vi "SP_Auto_Read_Write.vi"() -> ()   [LabVIEW 2013]
uses:
  <vilib>/event_ctls.llb/eventvkey.ctl
  Global_Not-Aus.vi
  Global_Start_Stop_Einzelschritt.vi
  <vilib>/Utility/file.llb/Write To Spreadsheet File (DBL).vi
  <vilib>/Utility/file.llb/Read From Spreadsheet File (string).vi
panel:
  in  "Multiple Control":T1(tab)
  out "P6":dbl[](array[numeric])
  out "P5":dbl[](array[numeric])
  out "P4":dbl[](array[numeric])
  out "P3":dbl[](array[numeric])
  out "P7":dbl[](array[numeric])
  out "P2":dbl[](array[numeric])
  out "P1":dbl[](array[numeric])
  out "P8":dbl[](array[numeric])
  out "P9":dbl[](array[numeric])
  out "P10":dbl[](array[numeric])
  in  "Z axis":enum16{"Up", "Down"}(ring)
  in  "Y axis":enum16{"Forward", "Backward"}(ring)
  in  "X axis":enum16{"Left", "Right"}(ring)
  in  "Move Steps":bool
  in  "Steps(mm)":dbl[](array[numeric]) min=0.0
  in  "Go To":bool
  in  "Position":T2(ring)
  in  "Save":bool
  in  "Reset All":bool
  in  "Reset":bool
  in  "Import":bool
  in  "Export":bool
  in  "File Path":path=path "Y:/01_Projekte/EPN93031_Schreibplatz/8_Konstruktionsunterlagen/8.5_Software/COPY_KOSY Steuerung LabVIEW/1.New_Code_2014_2015/2Pole_strip_Position.txt"
  out "Speed":dbl(knob) scale=0.0..10.0
  in  "Port for KOSY3":refnum<visa-resource-name>="COM2"
  in  "Port for Powersupply":refnum<visa-resource-name>="COM3"
  in  "Port for Write Head":refnum<visa-resource-name>="COM4"
  in  "Port for ED33":refnum<visa-resource-name>="COM7"
  in  "Port for ED32i":refnum<visa-resource-name>="COM8"
  in  "X,Y,Z Value Limits":T3={"mm Xmin "=0.0, "mm Xmax "=100.0, " mm Ymin "=0.0, "mm Ymax "=267.9, " mm Zmin"=0.0, "mm Zmax "=108.0, "Schritte oder mm Umin (0)"=0.0, "Schritte oder mm Umax (0)"=0.0, "Schritte oder mm Cmin (0)"=0.0, "Schritte oder mm Cmax (0)"=0.0, "Schritte oder mm Amin (0)"=0.0, "Schritte oder mm Amax (0)"=0.0, "Schritte oder mm Bmin (0)"=0.0, "Schritte oder mm Bmax (0)"=0.0}
  out "Error Out":errorcluster caption="error out"
  in  "Error In":errorcluster caption="error in"
  out "Movement":T4={"Axis"=36, "Direction(To/From)"=0, "Speed in mm/s\n (5)[0,025-20]"=5.0, "IV6"=FALSE} {"Direction(To/From)" items=["vom Endschalter weg", "zum Endschalter hin"]; "Speed in mm/s\n (5)[0,025-20]" min=0.025 max=20; "Axis" items=["X-Achse"=36, "Y-Achse"=37, "Z-Achse"=38, "U-Achse"=63]}
  out "Keyboard Press Display":cluster{"Speed(+/-)":i16, "Movement":T5}
  in  "Count":dbl
  in  "Move & Measure":bool
  in  "Clear Sensor Readings":bool
  in  "ED32i Active?":bool
  in  "ED33 Active?":bool
  in  "Stop Program":bool
  in  "Instructions":enum32{"Page 2"}(tab)
  in  "Main Tab":enum32{"Page 1", "Page 2"}(tab)
  in  "File Select":enum32{"Page 1"}(tab)
  out "Steps":dbl
  out "Current Sequence":string[](array[string])
  in  "Clear Sequence":bool
  in  "Load Sequence":bool
  out "Sequence":string[][](array[string])
  in  "File  Select":path
  in  "Activate Sequence?":bool
  in  "Results":enum32{"Page 1"}(tab)
  out "ED32i":cluster{"Array 4[0]":i32, "Array 4[1]":i32}(graph)
  out "ED33":i32[](graph)
  out "ED32i_output":string[][](array[string])
  out "ED33_output":string[][](array[string])
  in  "Home Position":bool
  out "Operation Done":string="Initialise"
  out "Current Status":string="Initialise"
  out "Moving":bool
  out "Stopped":bool
  out "Current Cordinates":T6 {"Schritte B" format="%#.4g"; "Schritte A" format="%#.4g"; "Schritte C" format="%#.4g"; "Schritte U" format="%#.4g"; "Z axis" format="%#.4g"; "Y axis" format="%#.4g"; "X axis" format="%#.4g"}
  # "Polestrip Positions"
  # "Com port info"
  # "Waveform Dispaly"
  # "Instructions\n                                              Manual Control\n1. Run the program.\n2. Select 'Initialise' to start the program from first \n     or 'Continue' to continue the ongoing process.\n3. Select 'Normal Operation'.\n\nPolestrip Positions\n1. If already positions are already saved, select the corresponding \n    file in 'File Path' and then click 'Import' to get the corresponding\n    positions displayed on the front panel. \n2. Set the 'Speed' using (+/-) for the movement.\n3. Select a position from the dropdown 'Position'and click 'Go To'.\n    Else, \n1. Set the 'Speed' using (+/-) for the movement.\n2. Set the length for movement in 'Steps(mm)'  in corresponding \n    axis and also the direction of travel in the selected axis. \n    Then press 'Move'.\n3. Once desired position is reached, select a position from the \n    dropdown 'Position' and click 'Save'.\n4. Once all positions are saved in front panel, select the file  to be \n     saved in 'File Path' and click 'Export' to save positions to a text file.\n5. Select a position from the dropdown 'Position' and \n    Click 'Reset' to clear individual position.\n6. Click 'Reset All' to clear all positions.\n \nSensor Readings\nContinuous measurement\n1.Activate the sensor to be read from 'Read Sensors' tab.\n2.Set the length for movement in 'Steps(mm)' in corresponding \n    axis and also the direction of travel in the selected axis. \n    Then press 'Move'.\nMove and Measure\n1. Activate the sensor to be read from 'Read Sensors' tab.\n2.Set 'Count' to the number of times to measure.\n2.Set the length for movement in 'Steps(mm)' in corresponding \n    axis and also the direction of travel in the selected axis. \n    Then press 'Move Measure'.\n\n1. Click 'Clear' in 'Read Sensors' tab to clear the sensor readings.\n\n                                          Automatic Execution\n1. Run the program.\n2. Select 'Initialise' to start the program from first \n     or 'Continue' to continue the ongoing process.\n3. Select 'Normal Operation'.\n4. Select the corresponding file in 'File Select' and then click 'Load' \n    to get the corresponding codes in 'Sequence' .\n5. Click 'Clear' to clear sequence.\n6. Click 'Activate Sequence?' to run the automatic execution. \n\n                                                       General\n1. Click 'Stop Program' to stop the running program.\n2. Click 'Home Position' to take the write head to (0,0,0)."
  # "Instructions\n\n\n1. Select the corresponding file in 'File Select' \n    and click 'Load' to get the codes in\n    'Sequence'.\n2. Click 'Clear' to clear sequence.\n3. Click 'Activate Sequence?' to run\n     the automatic execution."
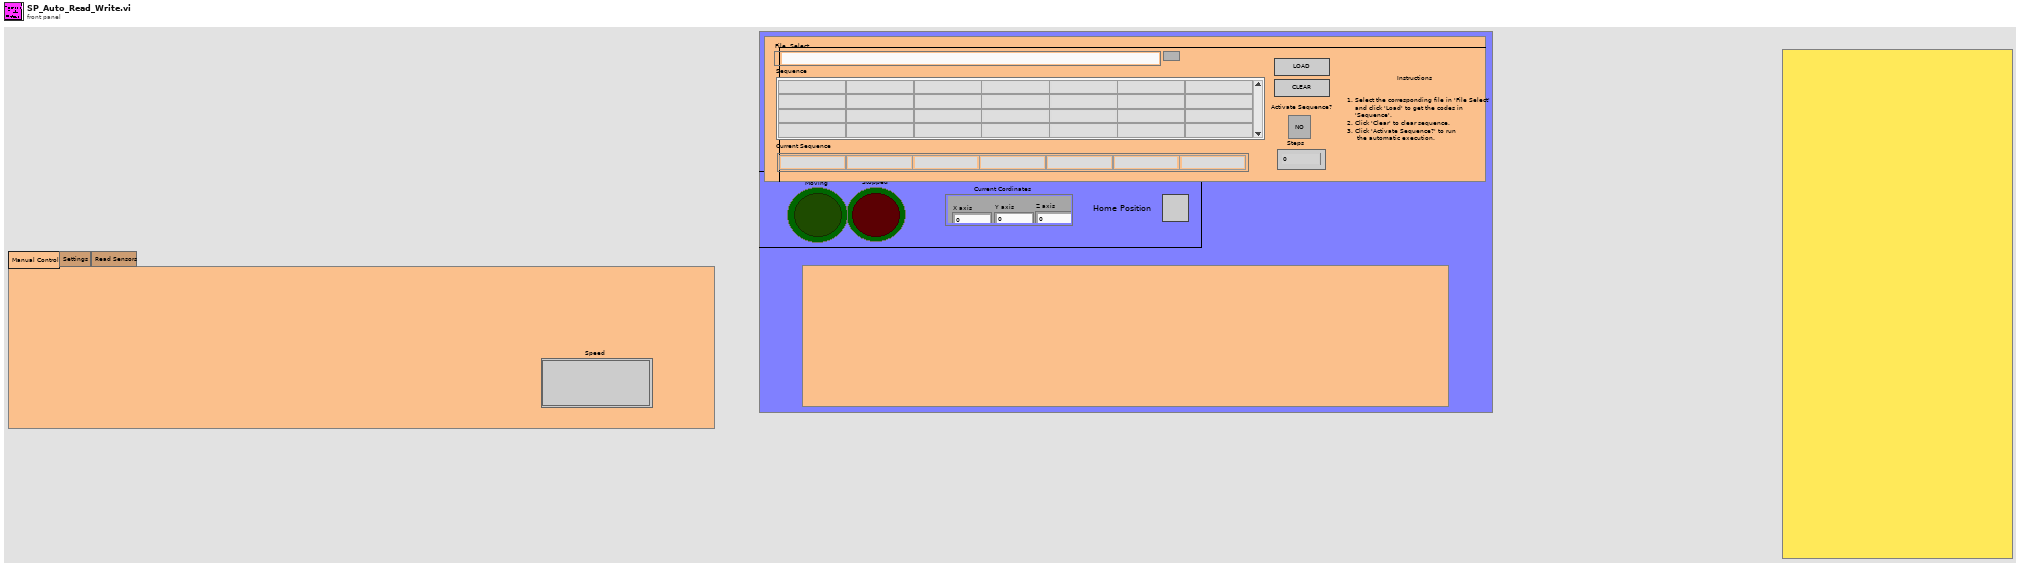
[diagram p1: front panel]
types:
  T1 = enum32{"Manual Control", "Settings", "Read Sensors"}
  T2 = enum16{"Position 1", "Position 2", "Position 3", "Position 4", "Position 5", "Position 6", "Position 7", "Position 8", "Position 9", "Position 10"}
  T3 = cluster{"mm Xmin ":sgl, "mm Xmax ":sgl, " mm Ymin ":sgl, "mm Ymax ":sgl, " mm Zmin":sgl, "mm Zmax ":sgl, "Schritte oder mm Umin (0)":sgl, "Schritte oder mm Umax (0)":sgl, "Schritte oder mm Cmin (0)":sgl, "Schritte oder mm Cmax (0)":sgl, "Schritte oder mm Amin (0)":sgl, "Schritte oder mm Amax (0)":sgl, "Schritte oder mm Bmin (0)":sgl, "Schritte oder mm Bmax (0)":sgl}
  T4 = cluster{"Axis":u8, "Direction(To/From)":u8, "Speed in mm/s\n (5)[0,025-20]":sgl, "IV6":bool}
  T5 = typedef "eventvkey.ctl" = enum16{"ASCII", "Enter", "Return", "Shift", "Ctrl", "Alt", "Cmd", "Opt", "Caps", "NumLock", "Clear", "Break", "Up", "Down", "Left", "Right", "Insert", "Delete", "Home", "End", "PageUp", "PageDown", "Escape", "Help", "Pause", "ScrollLock", "F1", "F2", "F3", "F4", "F5", "F6", "F7", "F8", "F9", "F10", "F11", "F12", "F13", "F14", "F15", "F16", "F17", "F18", "F19", "F20", "F21", "F22", "F23", "F24", "Play", "VolumeUp", "VolumeDown", "Mute", "Two Byte Char"}
  T6 = cluster{"X axis":sgl, "Y axis":sgl, "Z axis":sgl, "Schritte U":sgl, "Schritte C":sgl, "Schritte A":sgl, "Schritte B":sgl}
  T7 = enum32{"Page Enabled", "Page Disabled", "Page Disabled & Grayed"}
  T8 = cluster{"Geschwindigkeit X in mm/s\n(5) [0,025-15]":sgl, "Geschwindigkeit Y in mm/s\n(5) [0,025-15]":sgl, "Geschwindigkeit Z in mm/s\n(5) [0,025-15]":sgl, "GeschwindigkeitU in mm/s\n(5) [0,025-15]":sgl}
  T9 = cluster{"Schritte X":sgl, "Schritte Y":sgl, "Schritte Z":sgl, "Schritte U":sgl, "Schritte C":sgl, "Schritte A":sgl, "Schritte B":sgl}
  T10 = cluster{"[0]":dbl, "[1]":dbl, "[2]":dbl, "[3]":dbl, "[4]":dbl, "[5]":dbl, "[6]":dbl, "[7]":dbl, "[8]":dbl}
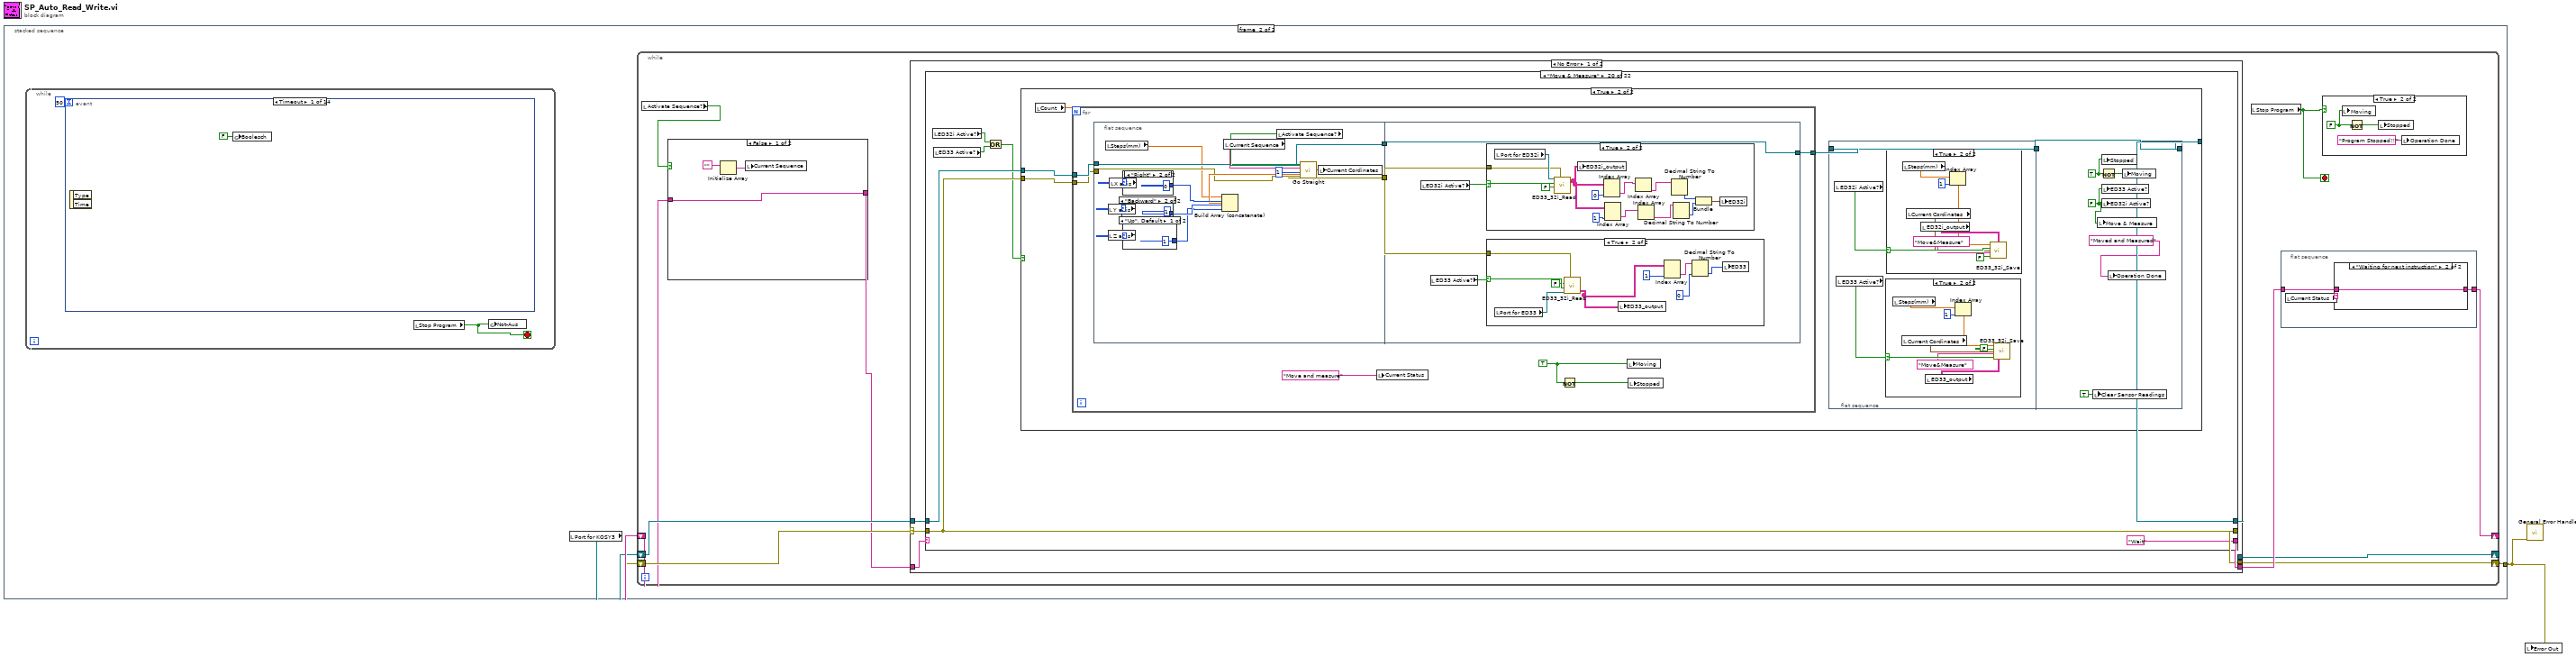
[diagram p0: block diagram]
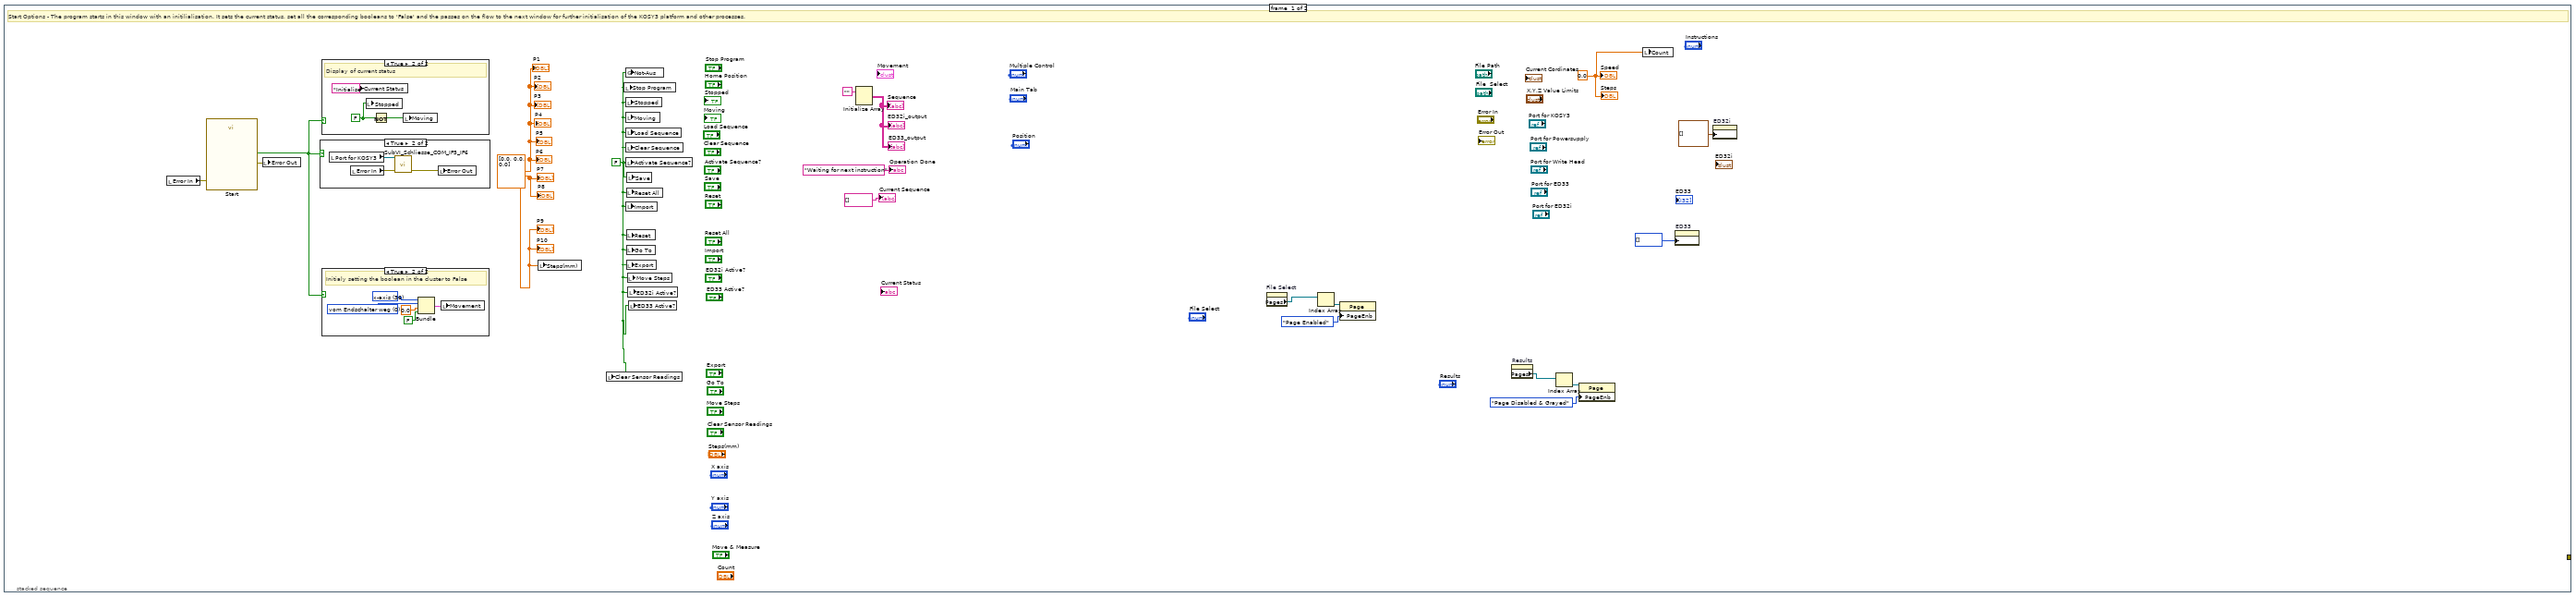
[diagram p2: hidden frame]
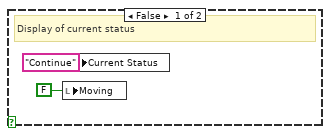
[diagram p5: hidden frame]
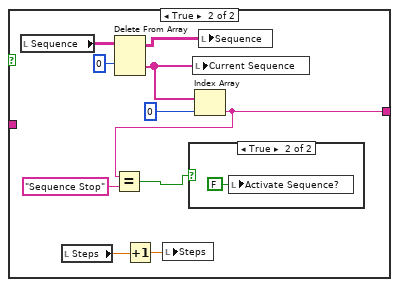
[diagram p6: hidden frame]
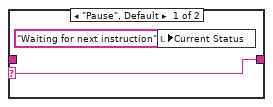
[diagram p9: hidden frame]
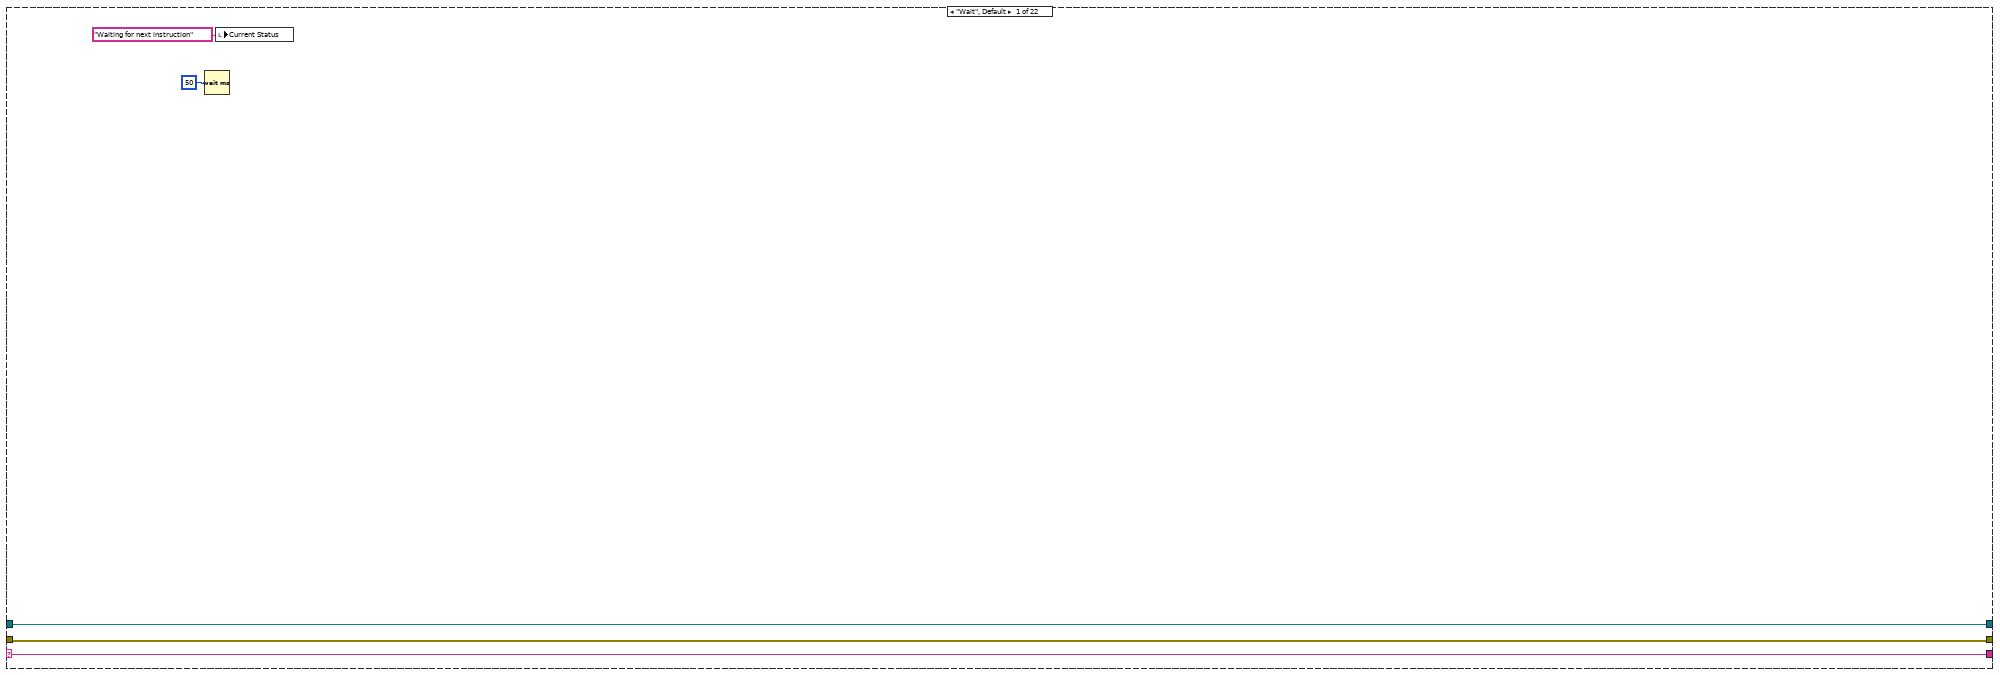
[diagram p10: hidden frame]
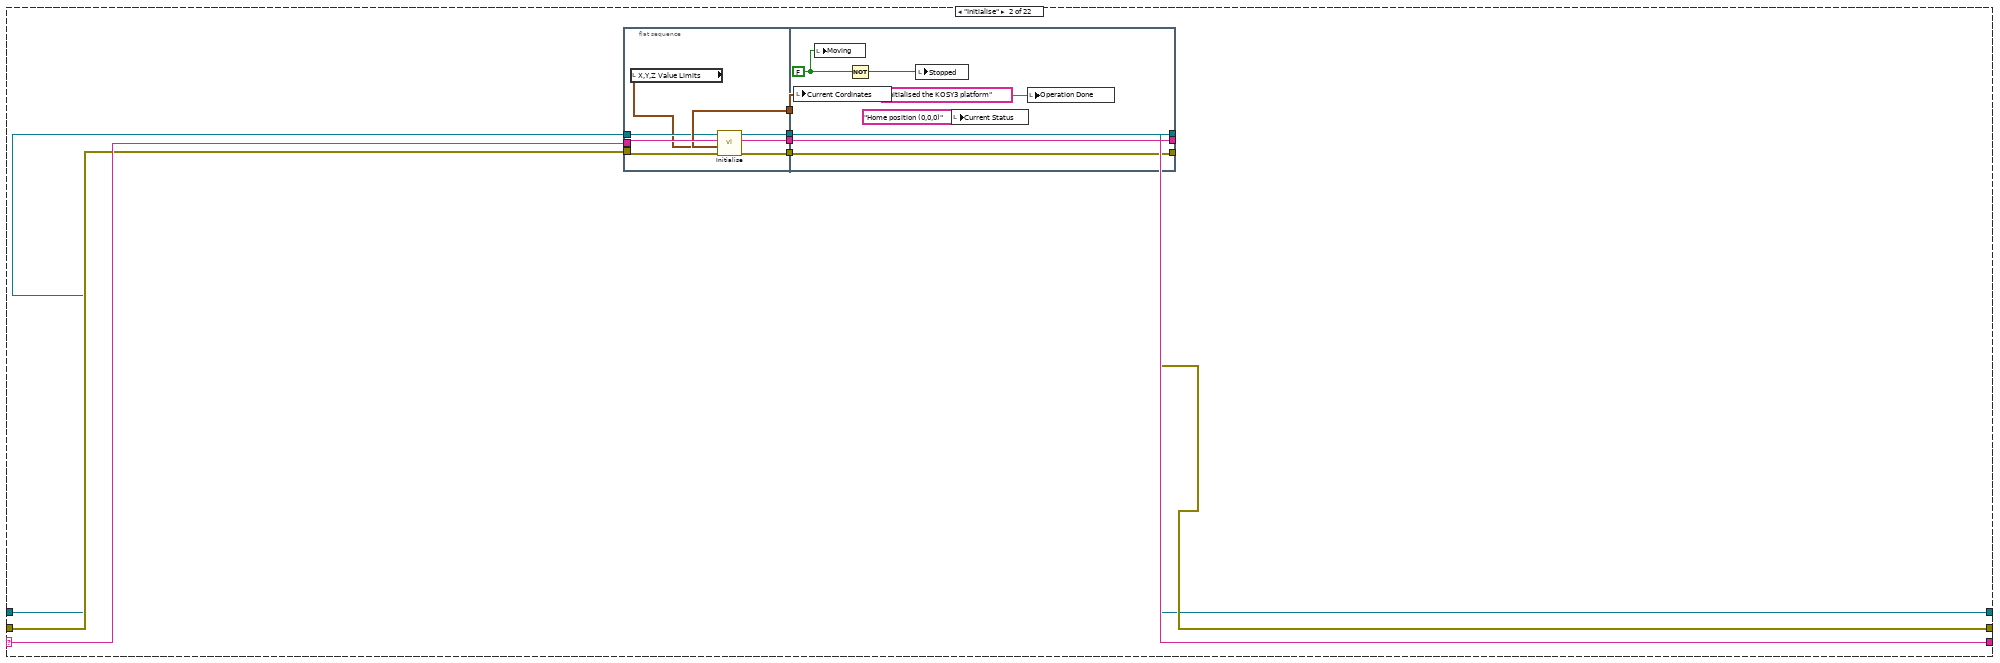
[diagram p11: hidden frame]
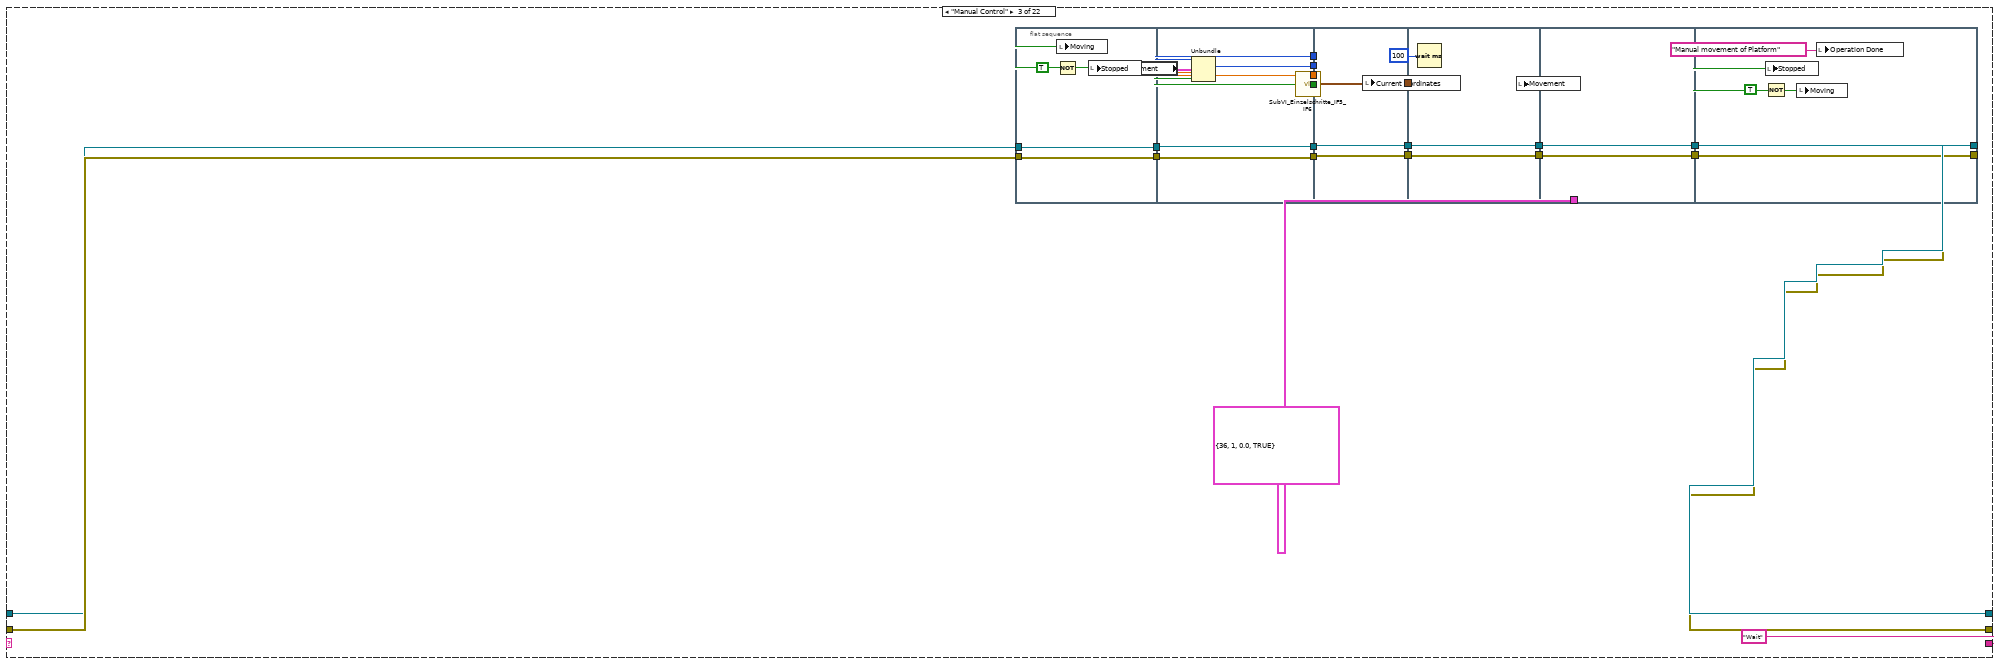
[diagram p12: hidden frame]
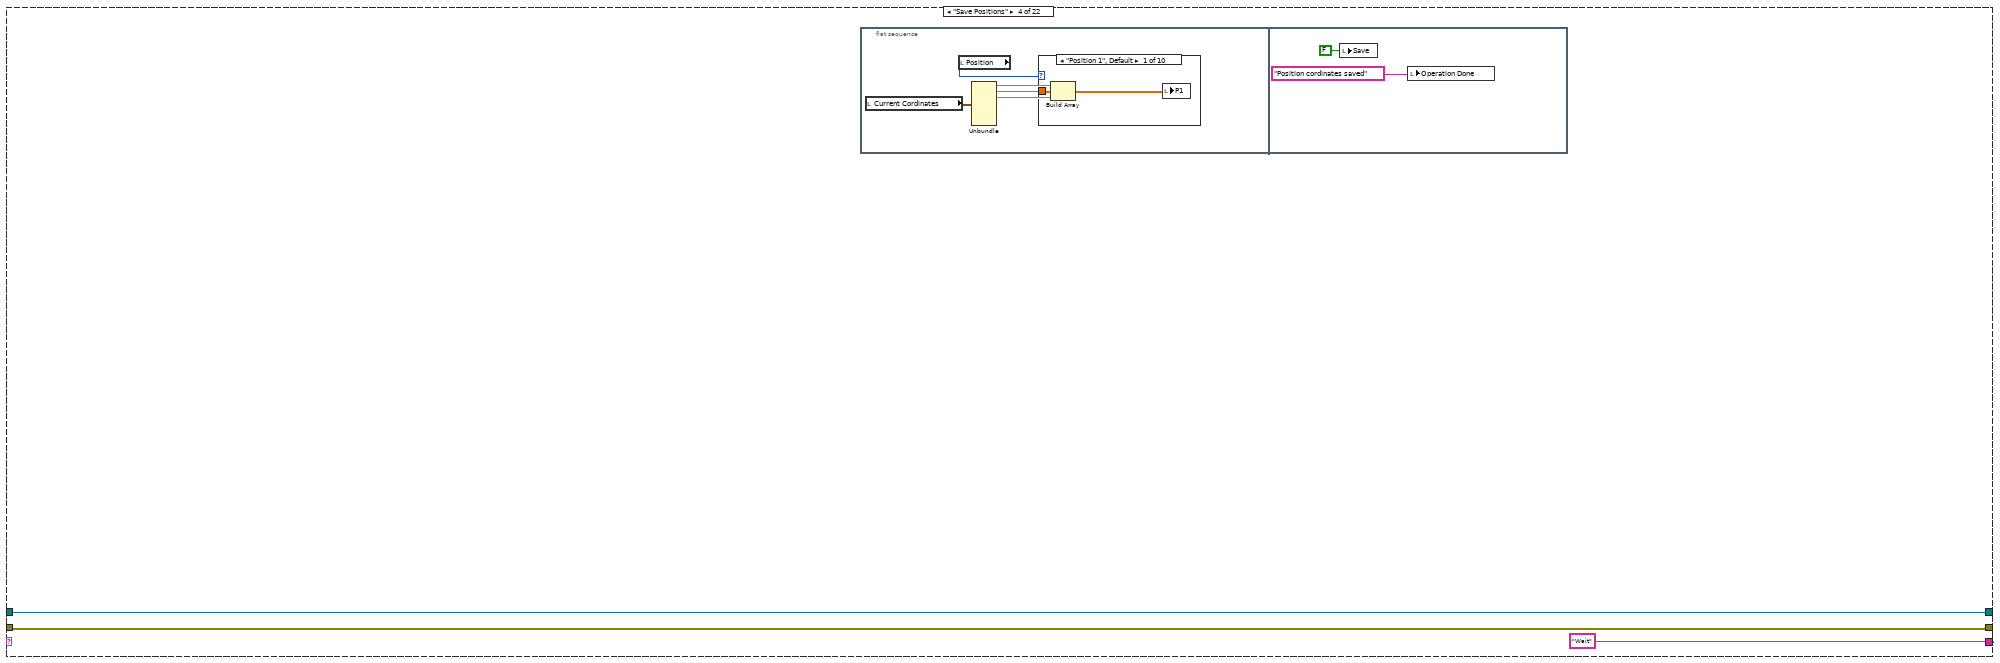
[diagram p13: hidden frame]
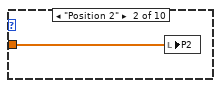
[diagram p14: hidden frame]
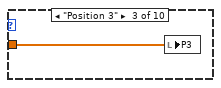
[diagram p15: hidden frame]
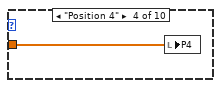
[diagram p16: hidden frame]
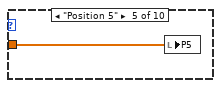
[diagram p17: hidden frame]
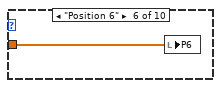
[diagram p18: hidden frame]
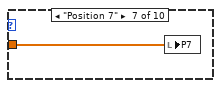
[diagram p19: hidden frame]
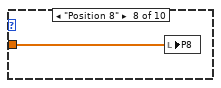
[diagram p20: hidden frame]
diagram:
  n1 = stacked-sequence {
    tunnel: [_ w33] -> w1
    frame #0 {
      w8 = 0.0 ("Speed")
      w9 = dbl[] [0.0, 0.0, 0.0] ("P1")
      w12 = FALSE ("Moving")
      # "Start Options - The program starts in this window with an initilialisation. It sets the current status, set all the corresponding booleans to 'False' and the passes on the flow to the next window for further initialisation of the KOSY3 platform and other processes."
      n2 = local read "Error In"() -> (w19:errorcluster)
      n3 = call "Start"("error in (no error)"=w19) -> ("Initialise"=w17:bool, "error out"=w18:errorcluster)  [unwired: 17 in]
      n4 = local write "Error Out"(w18) -> ()
      n5 = case shown="True" w17 {
        frame False {
        }
        frame True {
          n6 = local read "Port for KOSY3"() -> (w22:refnum<visa-resource-name>)
          n7 = local read "Error In"() -> (w21:errorcluster)
          n8 = call "SubVI_Schliesse_COM_IF5_IF6.vi"("VISA resource name in"=w22, "error in"=w21) -> ("error out"=w20:errorcluster)  [unwired: 13 in]
          n9 = local write "Error Out"(w20) -> ()
        }
      }
      n10 = case shown="True" w17 {
        frame False {
          # "Display of current status"
          n11 = local write "Moving"(FALSE ("Stopped")) -> ()
          n12 = local write "Current Status"("Continue") -> ()
        }
        frame True {
          w30 = FALSE ("Stopped")
          # "Display of current status"
          n13 = local write "Current Status"("Initialise") -> ()
          n14 = local write "Stopped"(w30) -> ()
          n15 = Not(x=w30) -> (.not. x?=w31:bool)
          n16 = local write "Moving"(w31) -> ()
        }
      }
      n17 = case shown="True" w17 {
        frame False {
        }
        frame True {
          w26 = u16 0 items=["vom Endschalter weg", "zum Endschalter hin"]
          w27 = u16 36 items=["x-axis"=36, "y-axis"=37, "z-axis"=38]
          # "Initialy setting the boolean in the cluster to False"
          n18 = Bundle(w27, w26, 0.0, FALSE) -> (w23:cluster{u16, u16, dbl, bool})  [unwired: 1 in]
          n19 = local write "Movement"(w23) -> ()
        }
      }
      n20 = local write "Steps(mm)"(w9) -> ()
      n21 = local write "Clear Sensor Readings"(w12) -> ()
      n22 = local write "Stop Program"(w12) -> ()
      n23 = global write "Global_Not-Aus.vi" "Not-Aus"(w12) -> ()
      n24 = local write "Stopped"(w12) -> ()
      n25 = local write "Moving"(w12) -> ()
      n26 = local write "Load Sequence"(w12) -> ()
      n27 = local write "Clear Sequence"(w12) -> ()
      n28 = local write "Activate Sequence?"(w12) -> ()
      n29 = local write "Import"(w12) -> ()
      n30 = local write "Reset All"(w12) -> ()
      n31 = local write "Reset"(w12) -> ()
      n32 = local write "Go To"(w12) -> ()
      n33 = local write "Export"(w12) -> ()
      n34 = local write "Save"(w12) -> ()
      n35 = local write "Move Steps"(w12) -> ()
      n36 = local write "ED32i Active?"(w12) -> ()
      n37 = local write "ED33 Active?"(w12) -> ()
      n38 = Initialize Array("" ("element")) -> (→"Sequence" →"ED32i_output" →"ED33_output":string[][])  [unwired: 2 in]
      n39 = property on="File Select" class="TabCtl (strict)"() -> ("Pages"=w2:refnum<vi>[])  [unwired: 2 in, 2 out]
      n40 = Index Array(array=w2) -> (element=w3:refnum<vi>)  [unwired: 1 in]
      n41 = property class="Page"(reference=w3, "PageEnb"=T7."Page Enabled" ("Page Enabled State")) -> ()  [unwired: 1 in, 2 out]
      n42 = property on="Results" class="TabCtl (strict)"() -> ("Pages"=w5:refnum<vi>[])  [unwired: 2 in, 2 out]
      n43 = Index Array(array=w5) -> (element=w6:refnum<vi>)  [unwired: 1 in]
      n44 = property class="Page"(reference=w6, "PageEnb"=T7."Page Disabled & Grayed" ("Page Enabled State")) -> ()  [unwired: 1 in, 2 out]
      n45 = local write "Count"(w8) -> ()
      n46 = property on="ED33" class="WFChart (strict)"("History Data"=i32[] []) -> ()  [unwired: 2 in, 2 out]
      n47 = property on="ED32i" class="WFChart (strict)"("History Data"=cluster{"Array 4[0]":i32, "Array 4[1]":i32}[] []) -> ()  [unwired: 2 in, 2 out]
      "Speed" <- w8
      "P1" <- w9
      "P2" <- w9
      "P3" <- w9
      "P7" <- w9
      "P4" <- w9
      "P5" <- w9
      "P6" <- w9
      "P8" <- w9
      "P9" <- w9
      "P10" <- w9
      "Current Sequence" <- string[] [] ("Current Sequence")
      "Operation Done" <- "Waiting for next instruction" ("Operation Done")
      "Steps" <- w8
    }
    frame #1 {
      n48 = while {
        stop <- w682 stop-if-true
        n49 = event shown="[0] Timeout" {
          selector: _ -> [_ _ _ _ _ _ _ _ _ _ _ _ _ _]
          dyn-events: _ -> [_ _ _ _ _ _ _ _ _ _ _ _ _ _]
          timeout: 50 -> [_ _ _ _ _ _ _ _ _ _ _ _ _ _]
          event Timeout {
            n50 = event-data() -> ()  [unwired: 1 in, 2 out]
            n51 = global write "Global_Start_Stop_Einzelschritt.vi" "Boolesch"(FALSE ("Boolesch")) -> ()
          }
          event Key Down? {
            # "This window checks for the key press in key board. Upon detection, it would set speed and (or) movement cluster and also updates the status."
            n52 = event-data() -> ("Char"=w684:i16, "VKey"=w686:T5)  [unwired: 1 in, 8 out]
            n53 = Wait (ms)(milliseconds to wait=u32 200) -> ()  [unwired: 1 out]
            n54 = Bundle("Char"=w684, "VKey"=w686) -> (→"Keyboard Press Display":cluster{"Char":i16, "VKey":T5})  [unwired: 1 in]
            n55 = local read "Moving"() -> (w688:bool)
            n56 = case shown="False" w688 {
              tunnel: w686 -> [w694 _]
              tunnel: w684 -> [w696 _]
              frame False {
                n57 = case shown="\"Return\", Default" w694 {
                  tunnel: [w697 w700 w703 w706 w709 w712 FALSE] -> w693
                  tunnel: [w699 w702 w705 w708 w711 w714 _] -> w691
                  tunnel: [w698 w701 w704 w707 w710 w713 _] -> w690
                  tunnel: TRUE -> [w697 w700 w703 w706 w709 w712 _]
                  frame "Left" {
                    w698 = u16 1 items=["vom Endschalter weg", "zum Endschalter hin"]
                    w699 = u16 36 items=["x-axis"=36, "y-axis"=37, "z-axis"=38]
                    # "Direction control(VKey identifies the directional keys)"
                  }
                  frame "Right" {
                    w701 = u16 0 items=["vom Endschalter weg", "zum Endschalter hin"]
                    w702 = u16 36 items=["x-axis"=36, "y-axis"=37, "z-axis"=38]
                    # "Direction control"
                  }
                  frame "Up" {
                    w704 = u16 1 items=["vom Endschalter weg", "zum Endschalter hin"]
                    w705 = u16 37 items=["x-axis"=36, "y-axis"=37, "z-axis"=38]
                    # "Direction control"
                  }
                  frame "Down" {
                    w707 = u16 0 items=["vom Endschalter weg", "zum Endschalter hin"]
                    w708 = u16 37 items=["x-axis"=36, "y-axis"=37, "z-axis"=38]
                  }
                  frame "PageUp" {
                    w710 = u16 1 items=["vom Endschalter weg", "zum Endschalter hin"]
                    w711 = u16 38 items=["x-axis"=36, "y-axis"=37, "z-axis"=38]
                  }
                  frame "PageDown" {
                    w713 = u16 0 items=["vom Endschalter weg", "zum Endschalter hin"]
                    w714 = u16 38 items=["x-axis"=36, "y-axis"=37, "z-axis"=38]
                  }
                  frame "Return", Default {
                  }
                }
                n58 = local read "Speed"() -> (w689:dbl)
                n59 = call "Speed_set.vi"("Speed"=w689, "Char"=w696) -> ("Speed"=w695:dbl)
                n60 = local write "Speed"(w695) -> ()
                n61 = case shown="True" w693 {
                  tunnel: w695 -> [_ w719]
                  tunnel: w691 -> [_ w718]
                  tunnel: w690 -> [_ w717]
                  frame False {
                  }
                  frame True {
                    n62 = Bundle(w718, w717, "Speed"=w719, TRUE) -> (w716:cluster{u16, u16, "Speed":dbl, bool})  [unwired: 1 in]
                    n63 = local write "Movement"(w716) -> ()
                    n64 = local write "Current Status"("Manual Control" ("Status")) -> ()
                  }
                }
              }
              frame True {
                n65 = global write "Global_Start_Stop_Einzelschritt.vi" "Boolesch"(TRUE) -> ()
                n66 = local write "Moving"(FALSE) -> ()
              }
            }
            n67 = event-data() -> ()  [unwired: 3 in, 1 out]
          }
          event "Home Position": Value Change {
            # "This window corresponds to the 'Home position' button on the Front Panel. Pressing the button will take KOSY3 paltform to the home position (0,0,0)"
            n68 = event-data() -> ()  [unwired: 1 in, 6 out]
            n69 = local write "Current Status"("Home Position" ("Status")) -> ()
          }
          event "Save": Value Change {
            # "When the 'SAVE' button in the Front Panel is pressed, it would save the current cordinates of the KOSY3 platform to the selected position."
            n70 = event-data() -> ()  [unwired: 1 in, 6 out]
            n71 = local write "Current Status"("Save Positions" ("Status")) -> ()
          }
          event "Reset": Value Change {
            # "When 'RESET' in the Front Panel is pressed, it resets the cordinates in the selected position to (0,0,0)"
            n72 = event-data() -> ()  [unwired: 1 in, 6 out]
            n73 = local write "Current Status"("Reset Position" ("Status")) -> ()
          }
          event "Reset All": Value Change {
            # "When 'RESET ALL' in the Front Panel is pressed, it resets the cordinates in all positions to (0,0,0)"
            n74 = event-data() -> ()  [unwired: 1 in, 6 out]
            n75 = local write "Current Status"("Reset All" ("Status")) -> ()
          }
          event "Go To": Value Change {
            n76 = event-data() -> ()  [unwired: 1 in, 6 out]
            n77 = local write "Current Status"("Go Position" ("Status")) -> ()
          }
          event "Move Steps": Value Change {
            n78 = event-data() -> ()  [unwired: 1 in, 6 out]
            n79 = local write "Current Status"("Go Straight" ("Status")) -> ()
          }
          event "Move & Measure": Value Change {
            n80 = event-data() -> ()  [unwired: 1 in, 6 out]
            n81 = local write "Current Status"("Move & Measure" ("Status")) -> ()
          }
          event "Import": Value Change {
            n82 = event-data() -> ()  [unwired: 1 in, 6 out]
            n83 = local write "Current Status"("Import Cordinates" ("Status")) -> ()
          }
          event "Export": Value Change {
            n84 = event-data() -> ()  [unwired: 1 in, 6 out]
            n85 = local write "Current Status"("Export Cordinates" ("Status")) -> ()
          }
          event "Load Sequence": Value Change {
            n86 = event-data() -> ()  [unwired: 1 in, 6 out]
            n87 = local write "Current Status"("Load Sequence" ("Status")) -> ()
          }
          event "Clear Sequence": Value Change {
            n88 = event-data() -> ()  [unwired: 1 in, 6 out]
            n89 = local write "Current Status"("Clear Sequence" ("Status")) -> ()
          }
          event "Clear Sensor Readings": Value Change {
            n90 = event-data() -> ()  [unwired: 1 in, 6 out]
            n91 = local write "Current Status"("Clear SensorReadings" ("Status")) -> ()
          }
        }
        n92 = local read "Stop Program"() -> (w682:bool)
        n93 = global write "Global_Not-Aus.vi" "Not-Aus"(w682) -> ()
      }
      n94 = local read "Port for KOSY3"() -> (w34:refnum<visa-resource-name>)
      n95 = local read "Current Status"() -> (w36:string)
      n96 = local read "Error In"() -> (w35:errorcluster)
      n97 = while {
        shift-right: [w40] -> w33
        shift-left: w35 -> [w46]
        shift-right: [w41] -> _
        shift-left: w34 -> [w42]
        shift-right: [w44] -> _
        shift-left: w36 -> [w39]
        stop <- w43 stop-if-true
        n98 = local read "Activate Sequence?"() -> (w37:bool)
        n99 = case shown="False" w37 {
          tunnel: w39 -> [w49 _]
          tunnel: [w49 w54] -> w38
          frame False {
            n100 = Initialize Array("") -> (w47:string[])  [unwired: 1 in]
            n101 = local write "Current Sequence"(w47) -> ()
          }
          frame True {
            n102 = local read "Sequence"() -> (w59:string[][])
            n103 = local read "Steps"() -> (w51:dbl)
            n104 = Delete From Array(array=w59, index (row)=0) -> (deleted portion=w56:string[], array with subset deleted=w57:string[][])  [unwired: 2 in]
            n105 = Increment(x=w51) -> (x+1=w50:dbl)
            n106 = local write "Steps"(w50) -> ()
            n107 = local write "Current Sequence"(w56) -> ()
            n108 = Index Array(array=w56, index=0) -> (element=w54:string)
            n109 = Equal?(x=w54, y="Sequence Stop") -> (x = y?=w52:bool)
            n110 = case shown="True" w52 {
              frame False {
              }
              frame True {
                n111 = local write "Activate Sequence?"(FALSE ("Activate Sequence?")) -> ()
              }
            }
            n112 = local write "Sequence"(w57) -> ()
          }
        }
        n113 = case shown="No Error" w46 {
          selector: w46 -> [w72 w676]
          tunnel: w38 -> [w75 _]
          tunnel: [w74 "Error" ("String 2")] -> w45
          tunnel: w42 -> [w73 w677]
          tunnel: [w70 w677] -> w41
          tunnel: [w71 w676] -> w40
          frame No Error {
            n114 = case shown="\"Move & Measure\"" w75 {
              selector: w75 -> [w79 w90 _ _ _ _ _ _ _ _ _ _ _ _ _ _ _ _ _ _ _ _]
              tunnel: [w79 w87 "Wait" "Wait" ("String 2") "Wait" ("String 2") "Wait" ("String 2") "Wait" ("String 2") "Wait" ("String 2") "Wait" ("String 2") "Wait" ("String 2") "Wait" ("String 2") "Wait" ("String 2") "Wait" ("String 2") "Wait" ("String 2") "Wait" ("String 2") "Wait" ("String 2") "Wait" ("String 2") "Wait" ("String 2") "Wait" ("String 2") "Wait" ("String 2") "Wait" ("String 2") "Wait" ("String 2")] -> w74
              tunnel: w73 -> [w76 w85 w115 w161 w182 w199 w209 w241 w257 w296 w319 w326 w335 w344 w353 w367 w402 w522 w551 w559 w661 w668]
              tunnel: w72 -> [w77 w86 w118 w160 w181 w198 w208 w242 w258 w298 w320 w327 w334 w345 w352 w368 w403 w520 w550 w560 w660 w670]
              tunnel: [w77 w83 w110 w160 w181 w198 w206 w242 w258 w293 w320 w327 w334 w345 w352 w369 w401 w520 w550 w560 w660 w669] -> w71
              tunnel: [w76 w81 w114 w161 w182 w199 w207 w241 w257 w295 w319 w326 w335 w344 w353 w370 w400 w522 w551 w558 w661 w668] -> w70
              frame "Wait", Default {
                n115 = Wait (ms)(milliseconds to wait=50) -> ()  [unwired: 1 out]
                n116 = local write "Current Status"("Waiting for next instruction" ("Status")) -> ()
              }
              frame "Initialise" {
                n117 = flat-sequence {
                  tunnel: w90 -> [w98]
                  tunnel: [w97] -> w89
                  tunnel: [w96] -> w88
                  tunnel: w86 -> [w95]
                  tunnel: w85 -> [w94]
                  tunnel: [w93] -> w84
                  tunnel: [w92] -> w82
                  tunnel: w89 -> [w103]
                  tunnel: w88 -> [w102]
                  tunnel: [w102] -> w87
                  tunnel: [w100] -> w81
                  tunnel: w84 -> [w100]
                  tunnel: [w99] -> w83
                  tunnel: w82 -> [w99]
                  frame #0 {
                    n118 = local read "X,Y,Z Value Limits"() -> (w91:T3)
                    n119 = call "Initialise.vi"("error IO"=w95, "X,Y,Z values"=w91, "String"=w98, "Port for KOSY3"=w94) -> ("Fehler (Ausgang)"=w92:errorcluster, "Cordinates of the  KOSY3 Platform"=w97:T9, "String 2"=w96:string, "VISA-Referenz (Ausgang)"=w93:refnum<visa-resource-name>)
                  }
                  frame #1 {
                    w104 = FALSE ("Stopped")
                    n120 = local write "Current Cordinates"(w103) -> ()
                    n121 = local write "Moving"(w104) -> ()
                    n122 = Not(x=w104) -> (.not. x?=w105:bool)
                    n123 = local write "Stopped"(w105) -> ()
                    n124 = local write "Current Status"("Home position (0,0,0)" ("Status")) -> ()
                    n125 = local write "Operation Done"("Initialised the KOSY3 platform" ("Operation Done")) -> ()
                  }
                }
              }
              frame "Manual Control" {
                n126 = flat-sequence {
                  tunnel: [w129] -> w119
                  tunnel: w118 -> [w129]
                  tunnel: [w128] -> w116
                  tunnel: w115 -> [w128]
                  tunnel: [w137] -> w126
                  tunnel: [w136] -> w125
                  tunnel: [w135] -> w124
                  tunnel: [w134] -> w123
                  tunnel: [w133] -> w120
                  tunnel: w119 -> [w133]
                  tunnel: [w132] -> w117
                  tunnel: w116 -> [w132]
                  tunnel: [w147] -> w122
                  tunnel: w126 -> [w146]
                  tunnel: w125 -> [w145]
                  tunnel: w124 -> [w144]
                  tunnel: w123 -> [w143]
                  tunnel: w120 -> [w142]
                  tunnel: w117 -> [w139]
                  tunnel: [w141] -> w111
                  tunnel: [w140] -> w107
                  tunnel: w122 -> [w150]
                  tunnel: [w149] -> w112
                  tunnel: w111 -> [w149]
                  tunnel: [w148] -> w108
                  tunnel: w107 -> [w148]
                  tunnel: cluster{u16, u16, dbl, bool} {36, 1, 0.0, TRUE} -> [w154]
                  tunnel: [w153] -> w113
                  tunnel: w112 -> [w153]
                  tunnel: [w152] -> w109
                  tunnel: w108 -> [w152]
                  tunnel: [w156] -> w114
                  tunnel: w113 -> [w156]
                  tunnel: [w155] -> w110
                  tunnel: w109 -> [w155]
                  frame #0 {
                    w130 = TRUE ("Moving")
                    n127 = Not(x=w130) -> (.not. x?=w131:bool)
                    n128 = local write "Moving"(w130) -> ()
                    n129 = local write "Stopped"(w131) -> ()
                  }
                  frame #1 {
                    n130 = local read "Movement"() -> (w138:T4)
                    n131 = Unbundle(w138) -> ("Axis"=w137:u8, "Direction(To/From)"=w136:u8, "Speed in mm/s\n (5)[0,025-20]"=w135:sgl, "IV6"=w134:bool)
                  }
                  frame #2 {
                    n132 = call <userlib>:"SubVI_Einzelschritte_IF5_IF6.vi"("VISA resource name in"=w139, "Achsen-Wahl (X)"=w146, "Geschwindigkeit\nin mm/s (5)[0,025-20]"=w144, "IF5=F/IF6=T\n(IF6=T) in"=w143, "error in"=w142, "Richtung (vEw)"=w145) -> ("VISA resource name out"=w141:refnum<visa-resource-name>, "Koordinaten IF6"=w147:T9, "error out"=w140:errorcluster)  [unwired: 3 in, 4 out]
                  }
                  frame #3 {
                    n133 = local write "Current Cordinates"(w150) -> ()
                    n134 = Wait (ms)(milliseconds to wait=u32 100) -> ()  [unwired: 1 out]
                  }
                  frame #4 {
                    n135 = local write "Movement"(w154) -> ()
                  }
                  frame #5 {
                    w159 = TRUE ("Moving")
                    n136 = Not(x=w159) -> (.not. x?=w158:bool)
                    n137 = local write "Stopped"(w159) -> ()
                    n138 = local write "Moving"(w158) -> ()
                    n139 = local write "Operation Done"("Manual movement of Platform" ("Status")) -> ()
                  }
                }
              }
              frame "Save Positions" {
                n140 = flat-sequence {
                  frame #0 {
                    n141 = local read "Current Cordinates"() -> (w166:T6)
                    n142 = local read "Position"() -> (w168:T2)
                    n143 = Unbundle(w166) -> ("X axis"=w163:sgl, "Y axis"=w164:sgl, "Z axis"=w165:sgl)  [unwired: 4 out]
                    n144 = Build Array(w163, w164, w165) -> (w167:sgl[])
                    n145 = case shown="\"Position 1\", Default" w168 {
                      tunnel: w167 -> [w169 w170 w171 w172 w173 w174 w175 w176 w177 w178]
                      frame "Position 1", Default {
                        n146 = local write "P1"(w169) -> ()
                      }
                      frame "Position 2" {
                        n147 = local write "P2"(w170) -> ()
                      }
                      frame "Position 3" {
                        n148 = local write "P3"(w171) -> ()
                      }
                      frame "Position 4" {
                        n149 = local write "P4"(w172) -> ()
                      }
                      frame "Position 5" {
                        n150 = local write "P5"(w173) -> ()
                      }
                      frame "Position 6" {
                        n151 = local write "P6"(w174) -> ()
                      }
                      frame "Position 7" {
                        n152 = local write "P7"(w175) -> ()
                      }
                      frame "Position 8" {
                        n153 = local write "P8"(w176) -> ()
                      }
                      frame "Position 9" {
                        n154 = local write "P9"(w177) -> ()
                      }
                      frame "Position 10" {
                        n155 = local write "P10"(w178) -> ()
                      }
                    }
                  }
                  frame #1 {
                    n156 = local write "Save"(FALSE ("Save Button")) -> ()
                    n157 = local write "Operation Done"("Position cordinates saved" ("Operation Done")) -> ()
                  }
                }
              }
              frame "Reset Position" {
                n158 = flat-sequence {
                  frame #0 {
                    n159 = local read "Position"() -> (w184:T2)
                    n160 = case shown="\"Position 10\"" w184 {
                      tunnel: dbl[] [0.0, 0.0, 0.0] ("P1") -> [w186 w187 w188 w189 w190 w191 w192 w193 w194 w195]
                      frame "Position 1", Default {
                        n161 = local write "P1"(w186) -> ()
                      }
                      frame "Position 2" {
                        n162 = local write "P2"(w187) -> ()
                      }
                      frame "Position 3" {
                        n163 = local write "P3"(w188) -> ()
                      }
                      frame "Position 4" {
                        n164 = local write "P4"(w189) -> ()
                      }
                      frame "Position 5" {
                        n165 = local write "P5"(w190) -> ()
                      }
                      frame "Position 6" {
                        n166 = local write "P6"(w191) -> ()
                      }
                      frame "Position 7" {
                        n167 = local write "P7"(w192) -> ()
                      }
                      frame "Position 8" {
                        n168 = local write "P8"(w193) -> ()
                      }
                      frame "Position 9" {
                        n169 = local write "P9"(w194) -> ()
                      }
                      frame "Position 10" {
                        n170 = local write "P10"(w195) -> ()
                      }
                    }
                  }
                  frame #1 {
                    n171 = local write "Reset"(FALSE ("Reset")) -> ()
                    n172 = local write "Operation Done"("The selected position is reset" ("Operation Done")) -> ()
                  }
                }
              }
              frame "Reset All" {
                n173 = flat-sequence {
                  frame #0 {
                    w201 = dbl[] [0.0, 0.0, 0.0] ("P1")
                    n174 = local write "P1"(w201) -> ()
                    n175 = local write "P2"(w201) -> ()
                    n176 = local write "P3"(w201) -> ()
                    n177 = local write "P4"(w201) -> ()
                    n178 = local write "P5"(w201) -> ()
                    n179 = local write "P6"(w201) -> ()
                    n180 = local write "P7"(w201) -> ()
                    n181 = local write "P8"(w201) -> ()
                    n182 = local write "P9"(w201) -> ()
                    n183 = local write "P10"(w201) -> ()
                    n184 = local write "Steps(mm)"(w201) -> ()
                  }
                  frame #1 {
                    n185 = local write "Reset All"(FALSE ("Reset all Positions")) -> ()
                    n186 = local write "Operation Done"("Reset all positions" ("Operation Done")) -> ()
                  }
                }
              }
              frame "Go Position" {
                n187 = flat-sequence {
                  tunnel: [w214] -> w205
                  tunnel: [w213] -> w204
                  tunnel: w209 -> [w216]
                  tunnel: w208 -> [w215]
                  tunnel: [w239] -> w206
                  tunnel: [w240] -> w207
                  tunnel: w205 -> [w240]
                  tunnel: w204 -> [w239]
                  frame #0 {
                    w212 = TRUE ("Moving")
                    n188 = local write "Moving"(w212) -> ()
                    n189 = local read "Position"() -> (w224:T2)
                    n190 = case shown="\"Position 10\"" w224 {
                      tunnel: [w225 w226 w227 w228 w229 w230 w231 w232 w233 w234] -> w222
                      frame "Position 1", Default {
                        n191 = local read "P1"() -> (w225:dbl[])
                      }
                      frame "Position 2" {
                        n192 = local read "P2"() -> (w226:dbl[])
                      }
                      frame "Position 3" {
                        n193 = local read "P3"() -> (w227:dbl[])
                      }
                      frame "Position 4" {
                        n194 = local read "P4"() -> (w228:dbl[])
                      }
                      frame "Position 5" {
                        n195 = local read "P5"() -> (w229:dbl[])
                      }
                      frame "Position 6" {
                        n196 = local read "P6"() -> (w230:dbl[])
                      }
                      frame "Position 7" {
                        n197 = local read "P7"() -> (w231:dbl[])
                      }
                      frame "Position 8" {
                        n198 = local read "P8"() -> (w232:dbl[])
                      }
                      frame "Position 9" {
                        n199 = local read "P9"() -> (w233:dbl[])
                      }
                      frame "Position 10" {
                        n200 = local read "P10"() -> (w234:dbl[])
                      }
                    }
                    n201 = Not(x=w212) -> (.not. x?=w211:bool)
                    n202 = local write "Stopped"(w211) -> ()
                    n203 = local read "Speed"() -> (w218:dbl)
                    n204 = local read "Current Cordinates"() -> (w221:T6)
                    n205 = Bundle(0, "Speed"=w218, 0) -> (w217:cluster{i32, "Speed":dbl, i32})  [unwired: 1 in]
                    n206 = call <userlib>:"SubVI_Punkt_anfahren_IF5_IF6.vi"("Angehängtes Array"=w222, "error in"=w215, "Koordinaten in IF6"=w221, "Geschwindigkeiten"=w217, "VISA resource name in"=w216) -> ("error out"=w213:errorcluster, "Koordinaten out IF6"=w223:T9, "VISA resource name in 2"=w214:refnum<visa-resource-name>)  [unwired: 1 in]
                    n207 = local write "Current Cordinates"(w223) -> ()
                  }
                  frame #1 {
                    w235 = TRUE ("Moving")
                    n208 = local write "Go To"(FALSE ("Go To")) -> ()
                    n209 = local write "Stopped"(w235) -> ()
                    n210 = Not(x=w235) -> (.not. x?=w236:bool)
                    n211 = local write "Moving"(w236) -> ()
                    n212 = local write "Operation Done"("Go to the selected position" ("Operation Done")) -> ()
                  }
                }
              }
              frame "Import Cordinates" {
                n213 = flat-sequence {
                  frame #0 {
                    n214 = local read "File Path"() -> (w254:path)
                    n215 = call "Dekoder Batch Speicher.vi"("Batchfeld Speicher"=w254) -> ("P9"=w244:dbl[], "P10"=w245:dbl[], "P1"=w246:dbl[], "P2"=w247:dbl[], "P8"=w248:dbl[], "P3"=w249:dbl[], "P4"=w250:dbl[], "P7"=w253:dbl[], "P6"=w251:dbl[], "P5"=w252:dbl[])  [unwired: 5 in]
                    n216 = local write "P9"(w244) -> ()
                    n217 = local write "P10"(w245) -> ()
                    n218 = local write "P1"(w246) -> ()
                    n219 = local write "P2"(w247) -> ()
                    n220 = local write "P8"(w248) -> ()
                    n221 = local write "P3"(w249) -> ()
                    n222 = local write "P4"(w250) -> ()
                    n223 = local write "P5"(w252) -> ()
                    n224 = local write "P6"(w251) -> ()
                    n225 = local write "P7"(w253) -> ()
                  }
                  frame #1 {
                    n226 = local write "Import"(FALSE ("Import")) -> ()
                    n227 = local write "Operation Done"("Import the position cordinates" ("Operation Done")) -> ()
                  }
                }
              }
              frame "Export Cordinates" {
                n228 = flat-sequence {
                  frame #0 {
                    n229 = Two Button Dialog(message="Copy the values to ? ", 1:"New File" ("F button name (\"Cancel\")"), 2:"Existing File" ("T button name (\"OK\")")) -> (T button?=w260:bool)
                    n230 = case shown="True" w260 {
                      frame False {
                        n231 = local read "P10"() -> (w270:dbl[])
                        n232 = local read "P1"() -> (w276:dbl[])
                        n233 = local read "P2"() -> (w275:dbl[])
                        n234 = local read "P3"() -> (w274:dbl[])
                        n235 = local read "P4"() -> (w273:dbl[])
                        n236 = local read "P5"() -> (w272:dbl[])
                        n237 = local read "P6"() -> (w271:dbl[])
                        n238 = local read "P7"() -> (w267:dbl[])
                        n239 = local read "P8"() -> (w268:dbl[])
                        n240 = local read "P9"() -> (w269:dbl[])
                        n241 = Build Array(w276, w275, w274, w273, w272, w271, w267, w268, w269, w270) -> (w264:dbl[][])
                        n242 = call-poly <vilib>:"Write To Spreadsheet File.vi"("format (%.3f)"="%.6f", "2D data"=w264) -> ("new file path (Not A Path if cancelled)"=w266:path)  [unwired: 6 in]
                        n243 = local write "File Path"(w266) -> ()
                      }
                      frame True {
                        n244 = local read "P10"() -> (w278:dbl[])
                        n245 = local read "P1"() -> (w279:dbl[])
                        n246 = local read "P2"() -> (w280:dbl[])
                        n247 = local read "P3"() -> (w281:dbl[])
                        n248 = local read "P4"() -> (w282:dbl[])
                        n249 = local read "P5"() -> (w283:dbl[])
                        n250 = local read "P6"() -> (w284:dbl[])
                        n251 = local read "P7"() -> (w285:dbl[])
                        n252 = local read "P8"() -> (w286:dbl[])
                        n253 = local read "P8"() -> (w287:dbl[])
                        n254 = Build Array(w279, w280, w281, w282, w283, w284, w285, w286, w287, w278) -> (w288:dbl[][])
                        n255 = local read "File Path"() -> (w277:path)
                        n256 = call-poly <vilib>:"Write To Spreadsheet File.vi"("format (%.3f)"="%.6f", "2D data"=w288, "file path (dialog if empty)"=w277) -> ()  [unwired: 5 in, 1 out]
                      }
                    }
                  }
                  frame #1 {
                    n257 = local write "Export"(FALSE ("Export")) -> ()
                    n258 = local write "Operation Done"("Export the position cordinates" ("Operation Done")) -> ()
                  }
                }
              }
              frame "Home Position" {
                n259 = flat-sequence {
                  tunnel: [w302] -> w299
                  tunnel: w298 -> [w302]
                  tunnel: [w301] -> w297
                  tunnel: w296 -> [w301]
                  tunnel: w299 -> [w309]
                  tunnel: w297 -> [w308]
                  tunnel: [w307] -> w294
                  tunnel: [w306] -> w292
                  tunnel: [w314] -> w295
                  tunnel: w294 -> [w314]
                  tunnel: [w313] -> w293
                  tunnel: w292 -> [w313]
                  frame #0 {
                    w303 = TRUE ("Moving")
                    n260 = Not(x=w303) -> (.not. x?=w304:bool)
                    n261 = local write "Moving"(w303) -> ()
                    n262 = local write "Stopped"(w304) -> ()
                  }
                  frame #1 {
                    w311 = u16 6 items=["X-Achse", "Y-Achse", "Z-Achse", "X- und Y-Achse", "X- und Z-Achse", "Y- und Z-Achse", "X, Y und Z-Achse", "U-Achse", "keine Achse"] ("Beteiligte Achsen (X,Y,Z,U)")
                    n263 = call "SubVI_Home_XYZU_IF5_IF6.vi"("VISA resource name in"=w308, "Beteiligte Achsen (X,Y,Z,U)"=w311, "Geschwindigkeiten"=T8 {"Geschwindigkeit X in mm/s\n(5) [0,025-15]"=10.0, "Geschwindigkeit Y in mm/s\n(5) [0,025-15]"=10.0, "Geschwindigkeit Z in mm/s\n(5) [0,025-15]"=10.0, "GeschwindigkeitU in mm/s\n(5) [0,025-15]"=2.0}, "IF5=F/IF6=T\n(IF6=T) in"=TRUE ("IF5=F/IF6=T\n(IF6=T) in"), "error in"=w309) -> ("VISA resource name out"=w307:refnum<visa-resource-name>, "Koordinaten IF6"=w310:T9, "error out"=w306:errorcluster)  [unwired: 3 in, 5 out]
                    n264 = local write "Current Cordinates"(w310) -> ()
                  }
                  frame #2 {
                    w317 = FALSE ("Moving")
                    n265 = Not(x=w317) -> (.not. x?=w318:bool)
                    n266 = local write "Moving"(w317) -> ()
                    n267 = local write "Stopped"(w318) -> ()
                    n268 = local write "Home Position"(FALSE ("Go To")) -> ()
                    n269 = local write "Operation Done"("The platform is taken to home position (0,0,0)" ("Operation Done")) -> ()
                  }
                }
              }
              frame "Load Sequence" {
                n270 = flat-sequence {
                  frame #0 {
                    n271 = local read "File  Select"() -> (w323:path)
                    n272 = call-poly <vilib>:"Read From Spreadsheet File.vi"("file path (dialog if empty)"=w323) -> ("all rows"=w322:string[][])  [unwired: 6 in, 4 out]
                    n273 = local write "Sequence"(w322) -> ()
                  }
                  frame #1 {
                    n274 = local write "Load Sequence"(FALSE ("Load Sequence")) -> ()
                    n275 = local write "Operation Done"("Sequence loaded" ("Status")) -> ()
                  }
                }
              }
              frame "Clear Sequence" {
                n276 = flat-sequence {
                  frame #0 {
                    n277 = Initialize Array("" ("element")) -> (w329:string[][])  [unwired: 2 in]
                    n278 = local write "Sequence"(w329) -> ()
                  }
                  frame #1 {
                    n279 = local write "Clear Sequence"(FALSE ("Clear Sequence")) -> ()
                    n280 = local write "Operation Done"("Sequence cleared" ("Status")) -> ()
                  }
                }
              }
              frame "Clear SensorReadings" {
                n281 = flat-sequence {
                  frame #0 {
                    n282 = local read "Clear Sensor Readings"() -> (w338:bool)
                    n283 = Initialize Array("" ("element")) -> (w339:string[][])  [unwired: 2 in]
                    n284 = local write "ED32i_output"(w339) -> ()
                    n285 = local write "ED33_output"(w339) -> ()
                    n286 = call "ED33_32i_Read.vi"("Clear"=w338) -> ()  [unwired: 5 in, 2 out]
                    n287 = property on="ED32i" class="WFChart (strict)"("History Data"=cluster{"Array 4[0]":i32, "Array 4[1]":i32}[] []) -> ()  [unwired: 2 in, 2 out]
                    n288 = property on="ED33" class="WFChart (strict)"("History Data"=i32[] []) -> ()  [unwired: 2 in, 2 out]
                  }
                  frame #1 {
                    n289 = local write "Clear Sensor Readings"(FALSE ("Clear Sensor Readings")) -> ()
                    n290 = local write "Operation Done"("Cleared sensor readings" ("Operation Done")) -> ()
                  }
                }
              }
              frame "Set Speed" {
                n291 = flat-sequence {
                  frame #0 {
                    n292 = local read "Current Sequence"() -> (w346:string[])
                    n293 = Index Array(array=w346, index=1) -> (element=w348:string)
                    n294 = Fract/Exp String To Number(string=w348) -> (number=w349:dbl)  [unwired: 3 in, 1 out]
                    n295 = local write "Speed"(w349) -> ()
                  }
                  frame #1 {
                    n296 = local write "Operation Done"("Speed Set") -> ()
                  }
                }
              }
              frame "Set Powersupply" {
                n297 = flat-sequence {
                  frame #0 {
                    n298 = local read "Current Sequence"() -> (w354:string[])
                    n299 = local read "Port for Powersupply"() -> (w360:refnum<visa-resource-name>)
                    n300 = Index Array(array=w354, index=1 ("Index")) -> (element=w356:string)
                    n301 = Concatenate Strings(w356, "\r") -> (w358:string)
                    n302 = call "Serial_com_powersupply für Funktion.vi"("VISA resource name"=w360, "write"=TRUE, "string to write"=w358) -> ()  [unwired: 6 in, 2 out]
                  }
                  frame #1 {
                    n303 = local read "Port for Write Head"() -> (w362:refnum<visa-resource-name>)
                    n304 = Concatenate Strings("GPV 6" ("string"), "\r") -> (w364:string)
                    n305 = call "Serial_com_powersupply für Funktion.vi"("VISA resource name"=w362, "write"=TRUE, "string to write"=w364) -> ()  [unwired: 6 in, 2 out]
                  }
                  frame #2 {
                    n306 = local write "Operation Done"("Powersupply Set") -> ()
                  }
                }
              }
              frame "Batch Position" {
                n307 = flat-sequence {
                  tunnel: [w375] -> w370
                  tunnel: [w374] -> w369
                  tunnel: w368 -> [w373]
                  tunnel: w367 -> [w372]
                  frame #0 {
                    n308 = local read "Current Sequence"() -> (w376:string[])
                    n309 = Index Array(array=w376, index=1) -> (element=w378:string)
                    n310 = case shown="\"Position 1\", Default" w378 {
                      tunnel: [w386 w387 w388 w389 w390 w391 w392 w393 w394 w395] -> w379
                      frame "Position 1", Default {
                        n311 = local read "P1"() -> (w386:dbl[])
                      }
                      frame "Position 2" {
                        n312 = local read "P2"() -> (w387:dbl[])
                      }
                      frame "Position 3" {
                        n313 = local read "P3"() -> (w388:dbl[])
                      }
                      frame "Position 4" {
                        n314 = local read "P4"() -> (w389:dbl[])
                      }
                      frame "Position 5" {
                        n315 = local read "P5"() -> (w390:dbl[])
                      }
                      frame "Position 6" {
                        n316 = local read "P6"() -> (w391:dbl[])
                      }
                      frame "Position 7" {
                        n317 = local read "P7"() -> (w392:dbl[])
                      }
                      frame "Position 8" {
                        n318 = local read "P8"() -> (w393:dbl[])
                      }
                      frame "Position 9" {
                        n319 = local read "P9"() -> (w394:dbl[])
                      }
                      frame "Position 10" {
                        n320 = local read "P10"() -> (w395:dbl[])
                      }
                    }
                    n321 = local read "Speed"() -> (w384:dbl)
                    n322 = Bundle(1, "Speed"=w384, 1) -> (w385:cluster{i32, "Speed":dbl, i32})  [unwired: 1 in]
                    n323 = local read "Current Cordinates"() -> (w380:T6)
                    n324 = call <userlib>:"SubVI_Punkt_anfahren_IF5_IF6.vi"("Angehängtes Array"=w379, "error in"=w373, "Koordinaten in IF6"=w380, "Geschwindigkeiten"=w385, "VISA resource name in"=w372) -> ("error out"=w374:errorcluster, "Koordinaten out IF6"=w381:T9, "VISA resource name in 2"=w375:refnum<visa-resource-name>)  [unwired: 1 in]
                    n325 = local write "Current Cordinates"(w381) -> ()
                  }
                  frame #1 {
                    n326 = local write "Operation Done"("Position Set") -> ()
                  }
                }
              }
              frame "Go Straight" {
                n327 = local read "ED32i Active?"() -> (w399:bool)
                n328 = local read "ED33 Active?"() -> (w398:bool)
                n329 = Or(x=w399, y=w398) -> (x .or. y?=w397:bool)
                n330 = case shown="True" w397 {
                  tunnel: w403 -> [w408 w440]
                  tunnel: w402 -> [w407 w443]
                  tunnel: [w406 w445] -> w401
                  tunnel: [w405 w442] -> w400
                  frame False {
                    n331 = flat-sequence {
                      tunnel: w408 -> [w422]
                      tunnel: [w424] -> w410
                      tunnel: [w423] -> w409
                      tunnel: w407 -> [w421]
                      tunnel: w410 -> [w438]
                      tunnel: [w438] -> w405
                      tunnel: [w437] -> w406
                      tunnel: w409 -> [w437]
                      frame #0 {
                        w428 = TRUE ("Moving")
                        n332 = local read "X axis"() -> (w417:enum16{"Left", "Right"})
                        n333 = local read "Y axis"() -> (w416:enum16{"Forward", "Backward"})
                        n334 = local read "Z axis"() -> (w415:enum16{"Up", "Down"})
                        n335 = case shown="\"Forward\", Default" w416 {
                          tunnel: [0 1] -> w419
                          frame "Forward", Default {
                          }
                          frame "Backward" {
                          }
                        }
                        n336 = case shown="\"Right\"" w417 {
                          tunnel: [1 0] -> w420
                          frame "Left", Default {
                          }
                          frame "Right" {
                          }
                        }
                        n337 = case shown="\"Down\"" w415 {
                          tunnel: [1 0] -> w418
                          frame "Up", Default {
                          }
                          frame "Down" {
                          }
                        }
                        n338 = local read "Steps(mm)"() -> (w414:dbl[])
                        n339 = local read "Current Sequence"() -> (w412:string[])
                        n340 = local read "Activate Sequence?"() -> (w426:bool)
                        n341 = Build Array (concatenate)(w414, w420, w419, w418) -> (w413:dbl[])
                        n342 = local read "Speed"() -> (w411:dbl)
                        n343 = Not(x=w428) -> (.not. x?=w427:bool)
                        n344 = local write "Moving"(w428) -> ()
                        n345 = local write "Stopped"(w427) -> ()
                        n346 = call "Go Straight.vi"("VISA resource name in"=w421, "Sequence Active"=w426, "array"=w412, "Speed"=w411, "Steps(mm)"=w413, "error in"=w422) -> ("VISA resource name out"=w424:refnum<visa-resource-name>, "Koordinaten IF6"=w425:T9, "error out"=w423:errorcluster)
                        n347 = local write "Current Cordinates"(w425) -> ()
                      }
                      frame #1 {
                        w439 = TRUE ("Stopped")
                        n348 = Not(x=w439) -> (.not. x?=w436:bool)
                        n349 = local write "Move Steps"(w436) -> ()
                        n350 = local write "Stopped"(w439) -> ()
                        n351 = local write "Moving"(w436) -> ()
                        n352 = local write "Operation Done"("Moved to corresponding position" ("Operation Done")) -> ()
                      }
                    }
                  }
                  frame True {
                    n353 = flat-sequence {
                      tunnel: w440 -> [w507]
                      tunnel: [w503] -> w444
                      tunnel: w443 -> [w502]
                      tunnel: [w501] -> w441
                      tunnel: [w519] -> w445
                      tunnel: w444 -> [w519]
                      tunnel: [w516] -> w442
                      tunnel: w441 -> [w516]
                      frame #0 {
                        w504 = TRUE ("Moving")
                        n354 = local read "Z axis"() -> (w498:enum16{"Up", "Down"})
                        n355 = local read "X axis"() -> (w500:enum16{"Left", "Right"})
                        n356 = local read "Y axis"() -> (w499:enum16{"Forward", "Backward"})
                        n357 = case shown="\"Backward\"" w499 {
                          tunnel: [0 1] -> w495
                          frame "Forward", Default {
                          }
                          frame "Backward" {
                          }
                        }
                        n358 = case shown="\"Right\"" w500 {
                          tunnel: [1 0] -> w496
                          frame "Left", Default {
                          }
                          frame "Right" {
                          }
                        }
                        n359 = case shown="\"Up\", Default" w498 {
                          tunnel: [1 0] -> w494
                          frame "Up", Default {
                          }
                          frame "Down" {
                          }
                        }
                        n360 = local read "Steps(mm)"() -> (w497:dbl[])
                        n361 = Build Array (concatenate)(w497, w496, w495, w494) -> (w493:dbl[])
                        n362 = local read "Activate Sequence?"() -> (w508:bool)
                        n363 = local read "Current Sequence"() -> (w509:string[])
                        n364 = call "Go Straight.vi"("VISA resource name in"=w502, "Sequence Active"=w508, "array"=w509, "Speed"=1, "Steps(mm)"=w493, "error in"=w507) -> ("VISA resource name out"=w501:refnum<visa-resource-name>, "Koordinaten IF6"=w506:T9, "error out"=w503:errorcluster)
                        n365 = Not(x=w504) -> (.not. x?=w505:bool)
                        n366 = local write "Moving"(w504) -> ()
                        n367 = local write "Current Cordinates"(w506) -> ()
                        n368 = local write "Stopped"(w505) -> ()
                      }
                      frame #1 {
                        w518 = TRUE ("Stopped")
                        n369 = Not(x=w518) -> (.not. x?=w517:bool)
                        n370 = local write "Stopped"(w518) -> ()
                        n371 = local write "Moving"(w517) -> ()
                        n372 = local write "Move Steps"(w517) -> ()
                      }
                    }
                    n373 = flat-sequence {
                      tunnel: w440 -> [w446]
                      frame #0 {
                        n374 = local read "ED32i Active?"() -> (w448:bool)
                        n375 = local read "ED33 Active?"() -> (w447:bool)
                        n376 = case shown="True" w448 {
                          selector: w448 -> [_ w450]
                          tunnel: w446 -> [_ w449]
                          frame False {
                          }
                          frame True {
                            n377 = while {
                              tunnel: w450 -> [w464]
                              tunnel: w449 -> [w463]
                              stop <- w462 stop-if-true
                              n378 = local read "Port for ED32i"() -> (w465:refnum<visa-resource-name>)
                              n379 = call "ED33_32i_Read.vi"("error in (no error)"=w463, "ED33 Active?"=FALSE, "ED32i Active?"=w464, "Port ED32i"=w465) -> ("ED32i_output"=w459:string[][])  [unwired: 2 in, 1 out]
                              n380 = local write "ED32i_output"(w459) -> ()
                              n381 = Index Array(array=w459, index (col)=0) -> (element=w458:string[])  [unwired: 1 in]
                              n382 = Index Array(array=w459, index (col)=1) -> (element=w456:string[])  [unwired: 1 in]
                              n383 = Index Array(array=w458) -> (element=w457:string)  [unwired: 1 in]
                              n384 = Index Array(array=w456) -> (element=w455:string)  [unwired: 1 in]
                              n385 = Decimal String To Number(string=w457) -> (number=w454:i32)  [unwired: 2 in, 1 out]
                              n386 = Decimal String To Number(string=w455) -> (number=w453:i32)  [unwired: 2 in, 1 out]
                              n387 = Bundle(w454, w453) -> (w452:cluster{i32, i32})  [unwired: 1 in]
                              n388 = local read "Stopped"() -> (w462:bool)
                              n389 = local write "ED32i"(w452) -> ()
                            }
                          }
                        }
                        n390 = case shown="True" w447 {
                          selector: w447 -> [_ w467]
                          tunnel: w446 -> [_ w466]
                          frame False {
                          }
                          frame True {
                            n391 = while {
                              tunnel: w467 -> [w475]
                              tunnel: w466 -> [w474]
                              stop <- w473 stop-if-true
                              n392 = local read "Port for ED33"() -> (w476:refnum<visa-resource-name>)
                              n393 = call "ED33_32i_Read.vi"("error in (no error)"=w474, "Port ED33"=w476, "ED33 Active?"=w475, "ED32i Active?"=FALSE) -> ("ED33_output"=w470:string[][])  [unwired: 2 in, 1 out]
                              n394 = local write "ED33_output"(w470) -> ()
                              n395 = Index Array(array=w470, index (col)=1) -> (element=w472:string[])  [unwired: 1 in]
                              n396 = Decimal String To Number(string=w472) -> (number=w469:i32[])  [unwired: 2 in, 1 out]
                              n397 = local read "Stopped"() -> (w473:bool)
                              n398 = local write "ED33"(w469) -> ()
                            }
                          }
                        }
                      }
                      frame #1 {
                        n399 = local read "ED32i Active?"() -> (w479:bool)
                        n400 = local read "ED33 Active?"() -> (w478:bool)
                        n401 = case shown="True" w479 {
                          selector: w479 -> [_ w483]
                          frame False {
                          }
                          frame True {
                            n402 = local read "Current Cordinates"() -> (w480:T6)
                            n403 = local read "ED32i_output"() -> (w482:string[][])
                            n404 = call "ED33_32i_Save.vi"("ED32i Active"=w483, "Cont/MM"="Continuous" ("Movement"), "ED33 Active?"=FALSE, "Current Cordinates"=w480, "ED32i_output"=w482) -> ()  [unwired: 2 in]
                          }
                        }
                        n405 = case shown="True" w478 {
                          selector: w478 -> [_ w487]
                          frame False {
                          }
                          frame True {
                            n406 = local read "Current Cordinates"() -> (w485:T6)
                            n407 = local read "ED33_output"() -> (w488:string[][])
                            n408 = call "ED33_32i_Save.vi"("ED32i Active"=FALSE, "Cont/MM"="Continuous" ("Movement"), "ED33 Active?"=w487, "Current Cordinates"=w485, "ED33_output"=w488) -> ()  [unwired: 2 in]
                          }
                        }
                        n409 = local write "Operation Done"("Read values from sensors and values saved" ("Operation Done")) -> ()
                      }
                      frame #2 {
                        w491 = FALSE ("ED32i Active?")
                        n410 = local write "ED32i Active?"(w491) -> ()
                        n411 = local write "ED33 Active?"(w491) -> ()
                        n412 = local write "Clear Sensor Readings"(TRUE ("Clear Sensor Readings")) -> ()
                      }
                    }
                  }
                }
              }
              frame "Set Steps" {
                n413 = flat-sequence {
                  frame #0 {
                    n414 = for {
                      N: 7 -> [_]
                      tunnel: [w543] -> w525 mode=indexing
                      i -> [w544]
                      n415 = local read "Current Sequence"() -> (w545:string[])
                      n416 = Increment(x=w544) -> (x+1=w547:i32)
                      n417 = Index Array(array=w545, index=w547) -> (element=w546:string)
                      n418 = Fract/Exp String To Number(string=w546) -> (number=w543:dbl)  [unwired: 3 in, 1 out]
                    }
                    n419 = Array To Cluster(array=w525) -> (cluster=w524:T10)
                    n420 = Unbundle(w524) -> ("[0]"=w526:dbl, "[1]"=w527:dbl, "[2]"=w528:dbl, "[3]"=w531:dbl, "[4]"=w532:dbl, "[5]"=w533:dbl)  [unwired: 3 out]
                    n421 = Bundle("[0]"=w526, "[1]"=w527, "[2]"=w528) -> (w529:cluster{"[0]":dbl, "[1]":dbl, "[2]":dbl})  [unwired: 1 in]
                    n422 = Cluster To Array(cluster=w529) -> (array=w530:dbl[])
                    n423 = case shown="1" w531 {
                      tunnel: [enum16{"Left", "Right"}."Right" enum16{"Left", "Right"}."Left"] -> w534
                      frame 0, Default {
                      }
                      frame 1 {
                      }
                    }
                    n424 = case shown="1" w532 {
                      tunnel: [enum16{"Forward", "Backward"}."Forward" enum16{"Forward", "Backward"}."Backward"] -> w536
                      frame 0, Default {
                      }
                      frame 1 {
                      }
                    }
                    n425 = case shown="1" w533 {
                      tunnel: [enum16{"Up", "Down"}."Down" enum16{"Up", "Down"}."Up"] -> w535
                      frame 0, Default {
                      }
                      frame 1 {
                      }
                    }
                    n426 = local write "Steps(mm)"(w530) -> ()
                    n427 = local write "X axis"(w534) -> ()
                    n428 = local write "Z axis"(w535) -> ()
                    n429 = local write "Y axis"(w536) -> ()
                  }
                  frame #1 {
                    n430 = local write "Operation Done"("Steps Set") -> ()
                  }
                }
              }
              frame "Set Count" {
                n431 = flat-sequence {
                  frame #0 {
                    n432 = local read "Current Sequence"() -> (w554:string[])
                    n433 = Index Array(array=w554, index=1) -> (element=w553:string)
                    n434 = Fract/Exp String To Number(string=w553) -> (number=w555:dbl)  [unwired: 3 in, 1 out]
                    n435 = local write "Count"(w555) -> ()
                  }
                  frame #1 {
                    n436 = local write "Operation Done"("Count Set") -> ()
                  }
                }
              }
              frame "Move & Measure" {
                n437 = local read "ED32i Active?"() -> (w562:bool)
                n438 = local read "ED33 Active?"() -> (w561:bool)
                n439 = Or(x=w562, y=w561) -> (x .or. y?=w557:bool)
                n440 = case shown="True" w557 {
                  tunnel: w559 -> [w564 w570]
                  tunnel: w560 -> [_ w569]
                  tunnel: [w564 w566] -> w558
                  frame False {
                  }
                  frame True {
                    n441 = local read "Count"() -> (w565:dbl)
                    n442 = for {
                      N: w565 -> [_]
                      tunnel: w570 -> [w603]
                      tunnel: w569 -> [w602]
                      tunnel: [w598] -> w567
                      w599 = TRUE
                      n443 = flat-sequence {
                        tunnel: w603 -> [w608]
                        tunnel: w602 -> [w607]
                        tunnel: [w606] -> w601
                        tunnel: [w605] -> w597
                        tunnel: w601 -> [w627]
                        tunnel: [w626] -> w598
                        tunnel: w597 -> [w626]
                        frame #0 {
                          n444 = local read "Steps(mm)"() -> (w604:dbl[])
                          n445 = local read "Y axis"() -> (w614:enum16{"Forward", "Backward"})
                          n446 = local read "Z axis"() -> (w615:enum16{"Up", "Down"})
                          n447 = local read "X axis"() -> (w616:enum16{"Left", "Right"})
                          n448 = case shown="\"Backward\"" w614 {
                            tunnel: [0 1] -> w618
                            frame "Forward", Default {
                            }
                            frame "Backward" {
                            }
                          }
                          n449 = case shown="\"Right\"" w616 {
                            tunnel: [1 0] -> w619
                            frame "Left", Default {
                            }
                            frame "Right" {
                            }
                          }
                          n450 = case shown="\"Up\", Default" w615 {
                            tunnel: [1 0] -> w617
                            frame "Up", Default {
                            }
                            frame "Down" {
                            }
                          }
                          n451 = Build Array (concatenate)(w604, w619, w618, w617) -> (w610:dbl[])
                          n452 = local read "Current Sequence"() -> (w611:string[])
                          n453 = local read "Activate Sequence?"() -> (w612:bool)
                          n454 = call "Go Straight.vi"("VISA resource name in"=w608, "Sequence Active"=w612, "array"=w611, "Speed"=1, "Steps(mm)"=w610, "error in"=w607) -> ("VISA resource name out"=w605:refnum<visa-resource-name>, "Koordinaten IF6"=w609:T9, "error out"=w606:errorcluster)
                          n455 = local write "Current Cordinates"(w609) -> ()
                        }
                        frame #1 {
                          n456 = local read "ED32i Active?"() -> (w629:bool)
                          n457 = local read "ED33 Active?"() -> (w628:bool)
                          n458 = case shown="True" w628 {
                            selector: w628 -> [_ w638]
                            tunnel: w627 -> [_ w636]
                            frame False {
                            }
                            frame True {
                              n459 = local read "Port for ED33"() -> (w637:refnum<visa-resource-name>)
                              n460 = call "ED33_32i_Read.vi"("error in (no error)"=w636, "Port ED33"=w637, "ED33 Active?"=w638, "ED32i Active?"=FALSE) -> ("ED33_output"=w633:string[][])  [unwired: 2 in, 1 out]
                              n461 = local write "ED33_output"(w633) -> ()
                              n462 = Index Array(array=w633, index (col)=1) -> (element=w635:string[])  [unwired: 1 in]
                              n463 = Decimal String To Number(string=w635, default (0L)=i64 0) -> (number=w632:i64[])  [unwired: 1 in, 1 out]
                              n464 = local write "ED33"(w632) -> ()
                            }
                          }
                          n465 = case shown="True" w629 {
                            selector: w629 -> [_ w652]
                            tunnel: w627 -> [_ w650]
                            frame False {
                            }
                            frame True {
                              n466 = local read "Port for ED32i"() -> (w651:refnum<visa-resource-name>)
                              n467 = call "ED33_32i_Read.vi"("error in (no error)"=w650, "ED33 Active?"=FALSE, "ED32i Active?"=w652, "Port ED32i"=w651) -> ("ED32i_output"=w641:string[][])  [unwired: 2 in, 1 out]
                              n468 = local write "ED32i_output"(w641) -> ()
                              n469 = Index Array(array=w641, index (col)=0) -> (element=w647:string[])  [unwired: 1 in]
                              n470 = Index Array(array=w641, index (col)=1) -> (element=w645:string[])  [unwired: 1 in]
                              n471 = Index Array(array=w647) -> (element=w646:string)  [unwired: 1 in]
                              n472 = Index Array(array=w645) -> (element=w644:string)  [unwired: 1 in]
                              n473 = Decimal String To Number(string=w646) -> (number=w643:i32)  [unwired: 2 in, 1 out]
                              n474 = Decimal String To Number(string=w644) -> (number=w642:i32)  [unwired: 2 in, 1 out]
                              n475 = Bundle(w643, w642) -> (w640:cluster{i32, i32})  [unwired: 1 in]
                              n476 = local write "ED32i"(w640) -> ()
                            }
                          }
                        }
                      }
                      n477 = local write "Current Status"("Move and measure") -> ()
                      n478 = Not(x=w599) -> (.not. x?=w600:bool)
                      n479 = local write "Moving"(w599) -> ()
                      n480 = local write "Stopped"(w600) -> ()
                    }
                    n481 = flat-sequence {
                      tunnel: [w571] -> w568
                      tunnel: w567 -> [w571]
                      tunnel: w568 -> [w593]
                      tunnel: [w593] -> w566
                      frame #0 {
                        n482 = local read "ED32i Active?"() -> (w573:bool)
                        n483 = local read "ED33 Active?"() -> (w572:bool)
                        n484 = case shown="True" w572 {
                          selector: w572 -> [_ w581]
                          frame False {
                          }
                          frame True {
                            n485 = local read "Steps(mm)"() -> (w575:dbl[])
                            n486 = local read "Current Cordinates"() -> (w577:T6)
                            n487 = local read "ED33_output"() -> (w579:string[][])
                            n488 = Index Array(array=w575, index=1) -> (element=w574:dbl)
                            n489 = call "ED33_32i_Save.vi"("Min_move"=w574, "ED32i Active"=FALSE, "Cont/MM"="Move&Measure" ("Movement"), "ED33 Active?"=w581, "Current Cordinates"=w577, "ED33_output"=w579) -> ()  [unwired: 1 in]
                          }
                        }
                        n490 = case shown="True" w573 {
                          selector: w573 -> [_ w589]
                          frame False {
                          }
                          frame True {
                            n491 = local read "Steps(mm)"() -> (w584:dbl[])
                            n492 = local read "Current Cordinates"() -> (w585:T6)
                            n493 = local read "ED32i_output"() -> (w587:string[][])
                            n494 = Index Array(array=w584, index=1) -> (element=w582:dbl)
                            n495 = call "ED33_32i_Save.vi"("Min_move"=w582, "ED32i Active"=w589, "Cont/MM"="Move&Measure" ("Movement"), "ED33 Active?"=FALSE, "Current Cordinates"=w585, "ED32i_output"=w587) -> ()  [unwired: 1 in]
                          }
                        }
                      }
                      frame #1 {
                        w595 = TRUE
                        w592 = FALSE
                        n496 = local write "Clear Sensor Readings"(TRUE ("Clear Sensor Readings")) -> ()
                        n497 = local write "Move & Measure"(w592) -> ()
                        n498 = Not(x=w595) -> (.not. x?=w594:bool)
                        n499 = local write "Stopped"(w595) -> ()
                        n500 = local write "ED33 Active?"(w592) -> ()
                        n501 = local write "ED32i Active?"(w592) -> ()
                        n502 = local write "Operation Done"("Moved and Measured") -> ()
                        n503 = local write "Moving"(w594) -> ()
                      }
                    }
                  }
                }
              }
              frame "Read Sensors" {
                n504 = flat-sequence {
                  frame #0 {
                    n505 = local read "Current Sequence"() -> (w664:string[])
                    n506 = Index Array(array=w664, index=1) -> (element=w662:string)
                    n507 = case shown="\"ED33\"" w662 {
                      frame "ED32i", Default {
                        n508 = local write "ED32i Active?"(TRUE ("ED32i Active?")) -> ()
                      }
                      frame "ED33" {
                        n509 = local write "ED33 Active?"(TRUE ("ED33 Active?")) -> ()
                      }
                    }
                  }
                  frame #1 {
                    n510 = local write "Operation Done"("Sensor selected") -> ()
                  }
                }
                n511 = property on="Results" class="TabCtl (strict)"() -> ("Pages"=w656:refnum<vi>[])  [unwired: 2 in, 2 out]
                n512 = property on="File Select" class="TabCtl (strict)"() -> ("Pages"=w653:refnum<vi>[])  [unwired: 2 in, 2 out]
                n513 = Index Array(array=w653) -> (element=w654:refnum<vi>)  [unwired: 1 in]
                n514 = Index Array(array=w656) -> (element=w657:refnum<vi>)  [unwired: 1 in]
                n515 = property class="Page"(reference=w654, "PageEnb"=T7."Page Disabled & Grayed" ("Page Enabled State")) -> ()  [unwired: 1 in, 2 out]
                n516 = property class="Page"(reference=w657, "PageEnb"=T7."Page Enabled" ("Page Enabled State")) -> ()  [unwired: 1 in, 2 out]
              }
              frame "Write Pole" {
                n517 = local read "Port for Powersupply"() -> (w671:refnum<visa-resource-name>)
                n518 = local read "Current Sequence"() -> (w673:string[])
                n519 = local read "Port for Write Head"() -> (w672:refnum<visa-resource-name>)
                n520 = call "Write Pole.vi"("Fehler (Eingang)"=w670, "array"=w673, "Port for write head"=w672, "Port for Powersupply"=w671) -> ("Fehler (Ausgang)"=w669:errorcluster)
              }
            }
          }
          frame Error {
            n521 = Unbundle(w676) -> ("source"=w675:string)  [unwired: 2 out]
            n522 = One Button Dialog(message=w675) -> (true=w679:bool)  [unwired: 1 in]
            n523 = local write "Stop Program"(w679) -> ()
            n524 = local write "Stopped"(w679) -> ()
            n525 = local write "Current Status"("Force stop due to error" ("Status")) -> ()
          }
        }
        n526 = local read "Stop Program"() -> (w43:bool)
        n527 = flat-sequence {
          tunnel: [w65] -> w44
          tunnel: w45 -> [w64]
          frame #0 {
            n528 = local read "Current Status"() -> (w66:string)
            n529 = case shown="\"Waiting for next instruction\"" w66 {
              selector: w66 -> [w68 _]
              tunnel: [w68 w69] -> w65
              tunnel: w64 -> [_ w69]
              frame "Pause", Default {
                n530 = local write "Current Status"("Waiting for next instruction" ("Status")) -> ()
              }
              frame "Waiting for next instruction" {
              }
            }
          }
        }
        n531 = case shown="True" w43 {
          frame False {
          }
          frame True {
            w61 = FALSE ("Moving")
            n532 = local write "Moving"(w61) -> ()
            n533 = Not(x=w61) -> (.not. x?=w62:bool)
            n534 = local write "Stopped"(w62) -> ()
            n535 = local write "Operation Done"("Program Stopped!!!" ("Status")) -> ()
          }
        }
      }
    }
  }
  n536 = local write "Error Out"(w1) -> ()
  n537 = call <vilib>:"General Error Handler.vi"("error in (no error)"=w1) -> ()  [unwired: 10 in, 5 out]
